vi "Demo Main.vi"() -> ()   [LabVIEW 2022 SP3]
uses:
  Logo.ctl
  C:/Users/Public/OneDrive/Desktop/PMT program/SampleCodeLabView/Kinesis_with_LabVIEW_Examples_LV12 - v3/Thorlabs.MotionControl.Controls.dll
  Kinesis_with_LabVIEW_Examples_LV12 - v3/Thorlabs.MotionControl.Controls.dll
  <vilib>/Utility/file.llb/Write Delimited Spreadsheet (string).vi
  <vilib>/Utility/file.llb/Write Delimited Spreadsheet (I64).vi
  <vilib>/Utility/file.llb/Write Delimited Spreadsheet (DBL).vi
  C:/Users/Public/OneDrive/Desktop/PMT program/SampleCodeLabView/Kinesis_with_LabVIEW_Examples_LV12 - v3/ThorLabs.MotionControl.KCube.DCServoCLI.dll
  Kinesis_with_LabVIEW_Examples_LV12 - v3/ThorLabs.MotionControl.KCube.DCServoCLI.dll
  <vilib>/Analysis/NI_AALBase.lvlib
panel:
  out "Polar Plot":picture
  in  "Wait to Start (ms)":i32
  in  "Laser Power (mW)":string="sample"
  in  "Sample Name":string="sample"
  in  "Save All Gate Data":bool
  out "ESD":i32=10000 caption="Steps\nAdded/Removed"
  in  "ES":i32 caption="Add /Remove \nSteps"
  out "Sweep Graph":u32[](graph)
  out "SM":i32 caption="Sweep\nMean"
  out "SN":i32 caption="Current Sweep Iteration"
  out "SND":i32 caption="Total No. of Sweeps"
  in  "Auto-Sweep":bool
  in  "P8":bool
  out "PC":i32 caption="Current \nPosition"
  out "WTD":i32=10000 caption="Wait Time (ms)\nRead Data"
  out "EPD":i32 caption="End Position\nRead Data"
  out "SPD":i32 caption="Start Position\nRead Data"
  out "SSD":i32 caption="Step Size\nRead Data"
  in  "SP":i32 caption="Start Position (degrees)\n Set Data"
  in  "WT":i32=10000 caption="Wait Time (ms)\n Set Data"
  in  "EP":i32 caption="End Position (degrees)\n Set Data"
  in  "P7":bool
  in  "SS":i32 caption="Step Size (degrees)\nSet Data"
  in  "Motor Controller\nSerialNumber":string="27261255"
  in  "KCubeDCServoControl":refnum<k24>(container)
  in  "Export":bool
  out "DB":u32[](array[numeric])
  out "OVL":bool caption="LED ON : Over Rang Data"
  out "OLD":i32
  out "GN":i32 caption="Gate Number"
  in  "Correction":bool=TRUE
  in  "Logo":T1
  out "Graph":u32[](graph)
  in  "Stop":bool
  in  "Start":bool
  in  "P6":bool
  out "RND":i32 caption="Read Number\nRead Data"
  in  "P5":bool
  in  "RN":i32=100 caption="Read Number\nSet Data"
  out "PowerD":i32 caption="Power\nRead Data"
  out "ITD":i32 caption="Internal Time\nRead Data"
  in  "P4":bool
  in  "P3":bool
  in  "IT":i32=100 caption="Internal Time\nSet Data"
  in  "P2":bool
  out "Handle Number":i32
  in  "P1":bool caption="Switch\nPower OFF/Power ON"
  in  "EXIT":bool
  # "pmt serial: 30430219"
  # "note: If you change angle between linear polarized light and half-wave plate by theta, the \npolarization after the wave plate is changed by twice theta. The code doesn't account for this.\nThis means we really need to go only to 180degrees, because at that point we have rotated the polarization by 360deg."
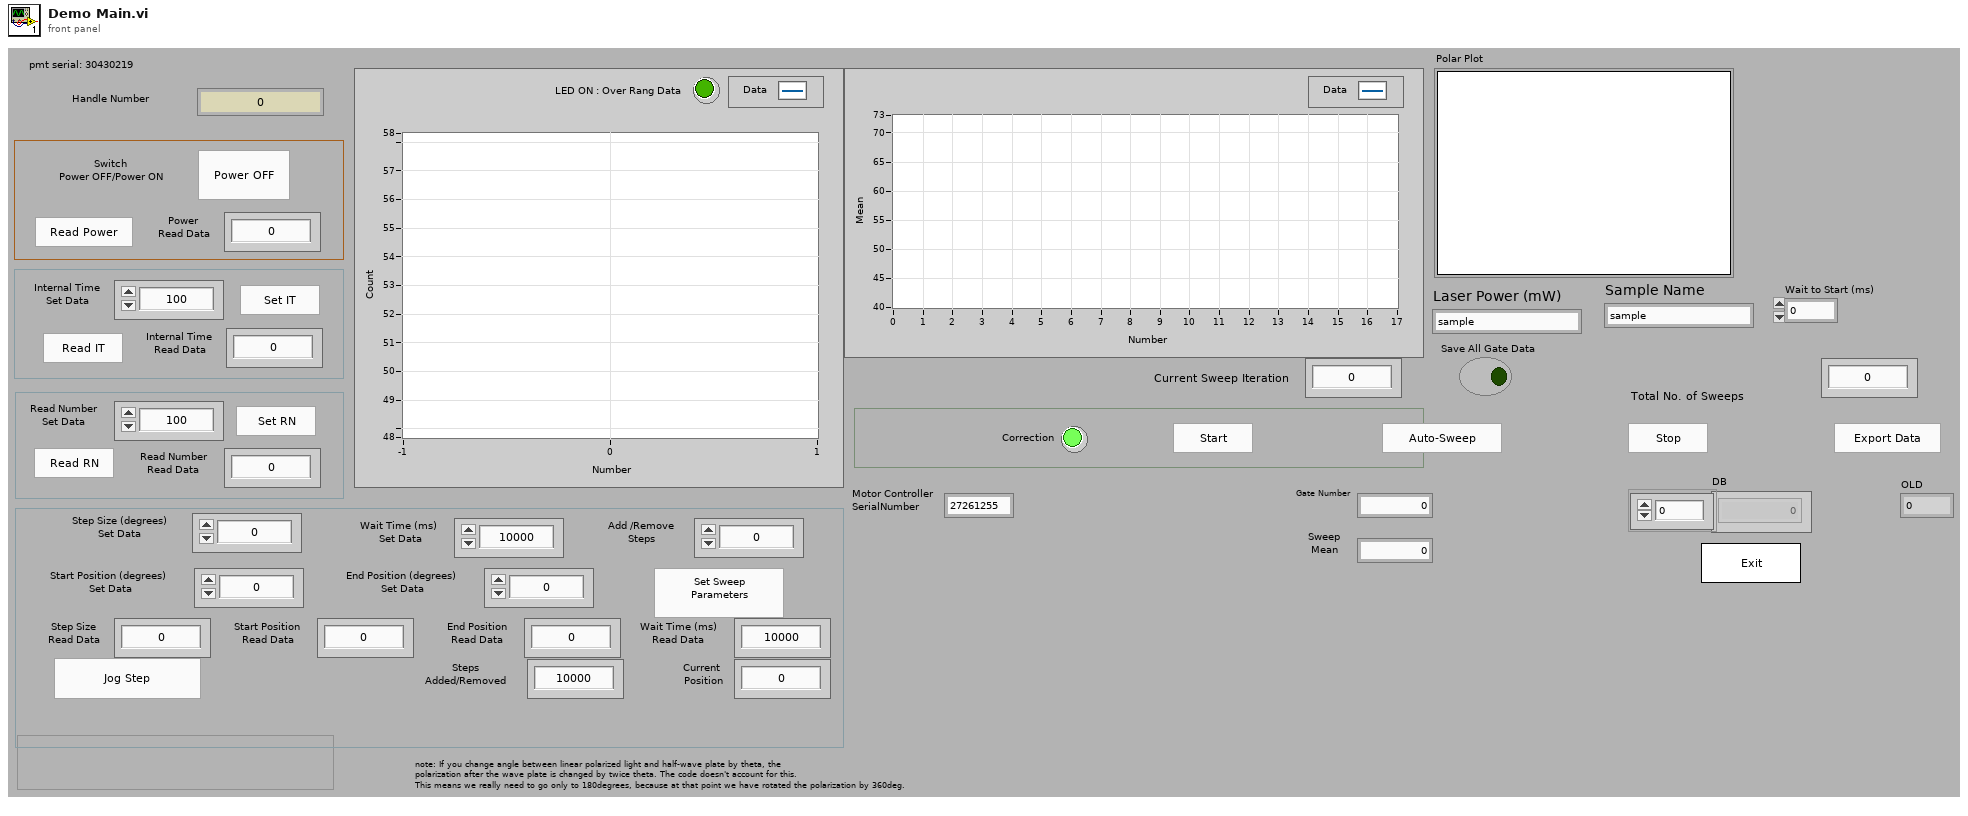
[diagram p1: front panel]
types:
  T1 = typedef "Logo.ctl" = bool
  T2 = enum8{"Enabled", "Disabled", "Disabled and Grayed Out"}
  T3 = typedef "LVBoundsTypeDef.ctl" = cluster{"Width":u32, "Height":u32}
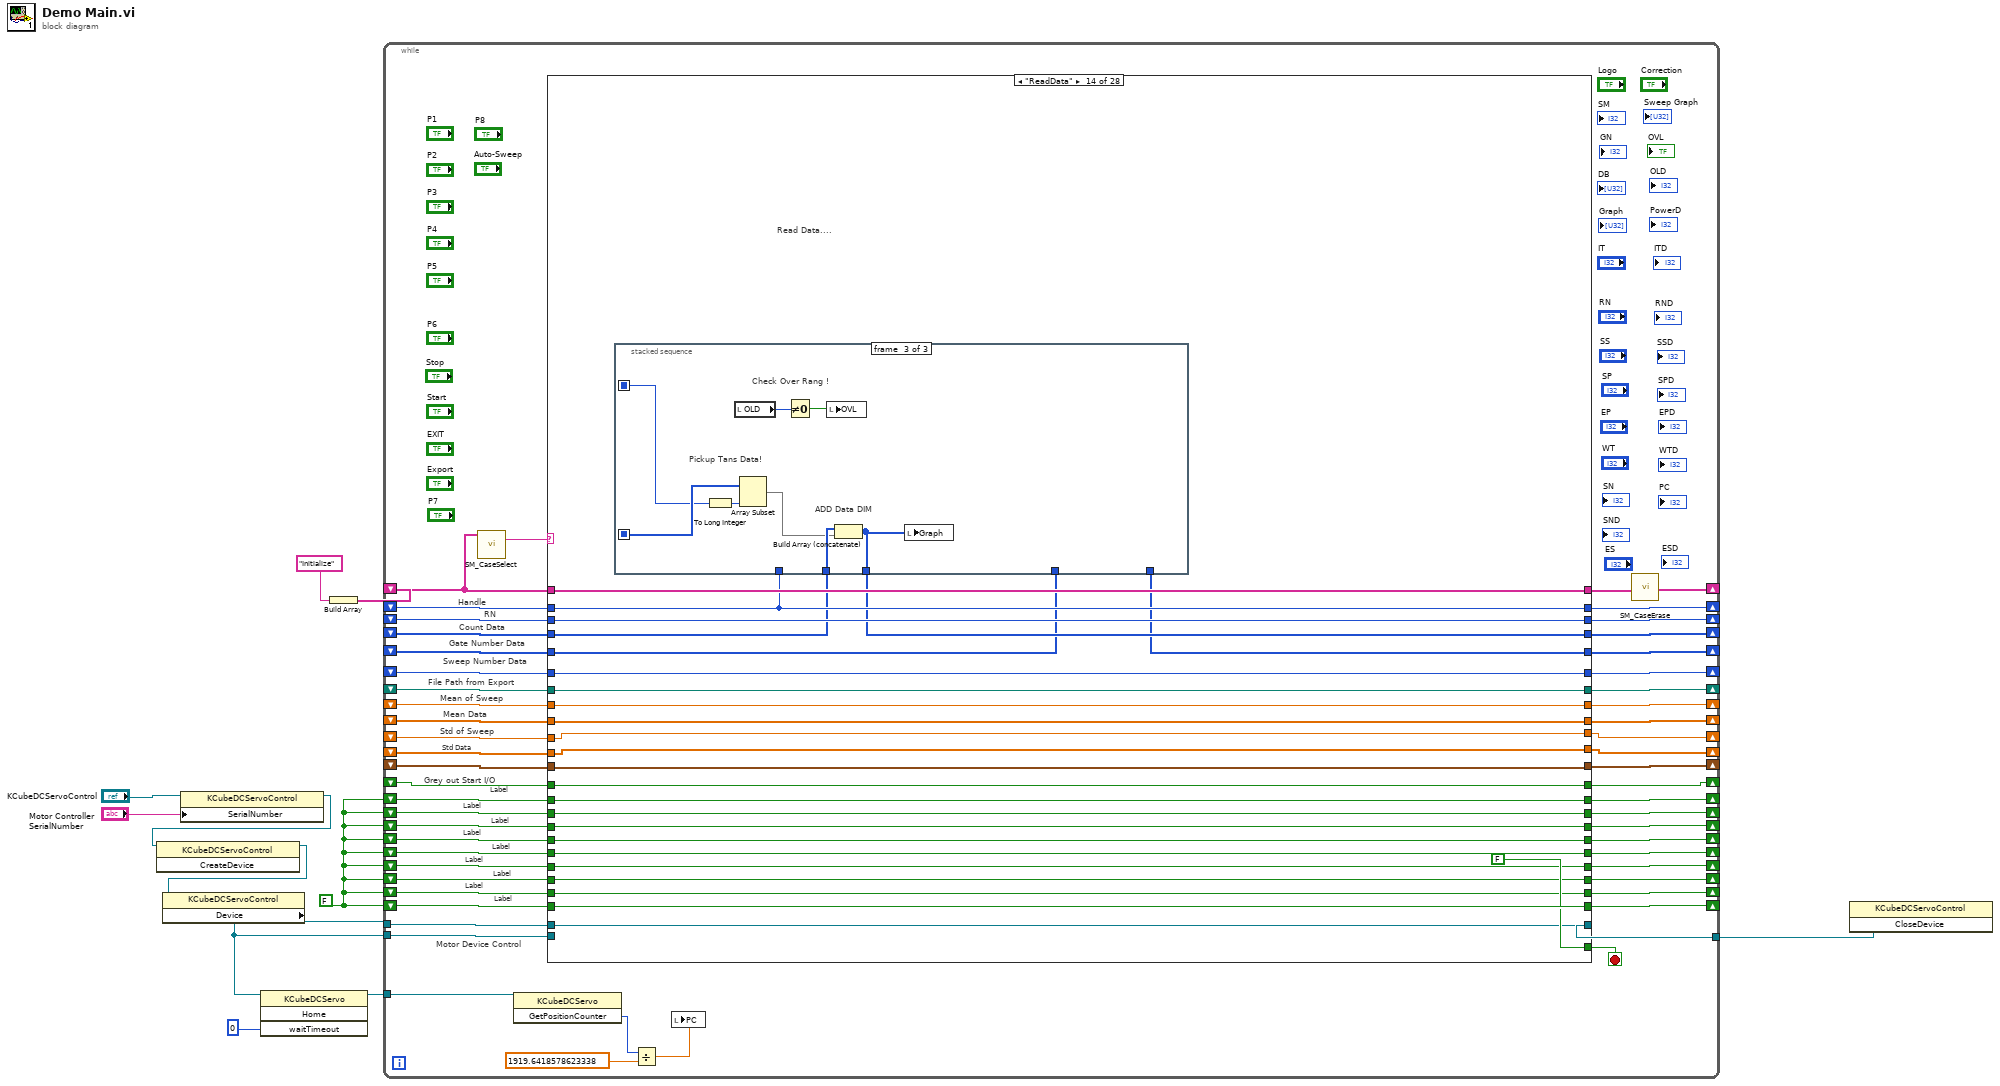
[diagram p0: block diagram]
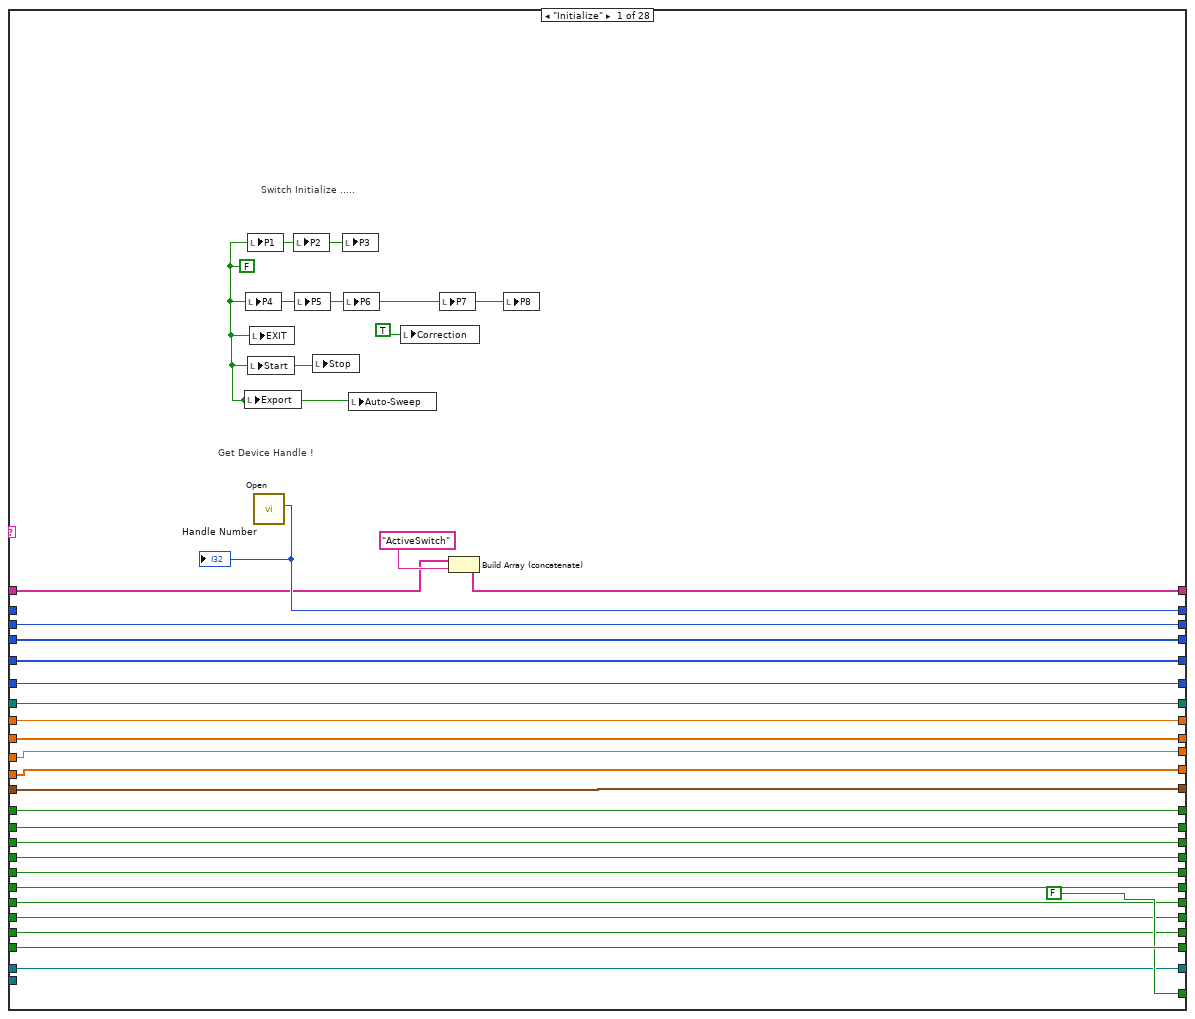
[diagram p2: hidden frame]
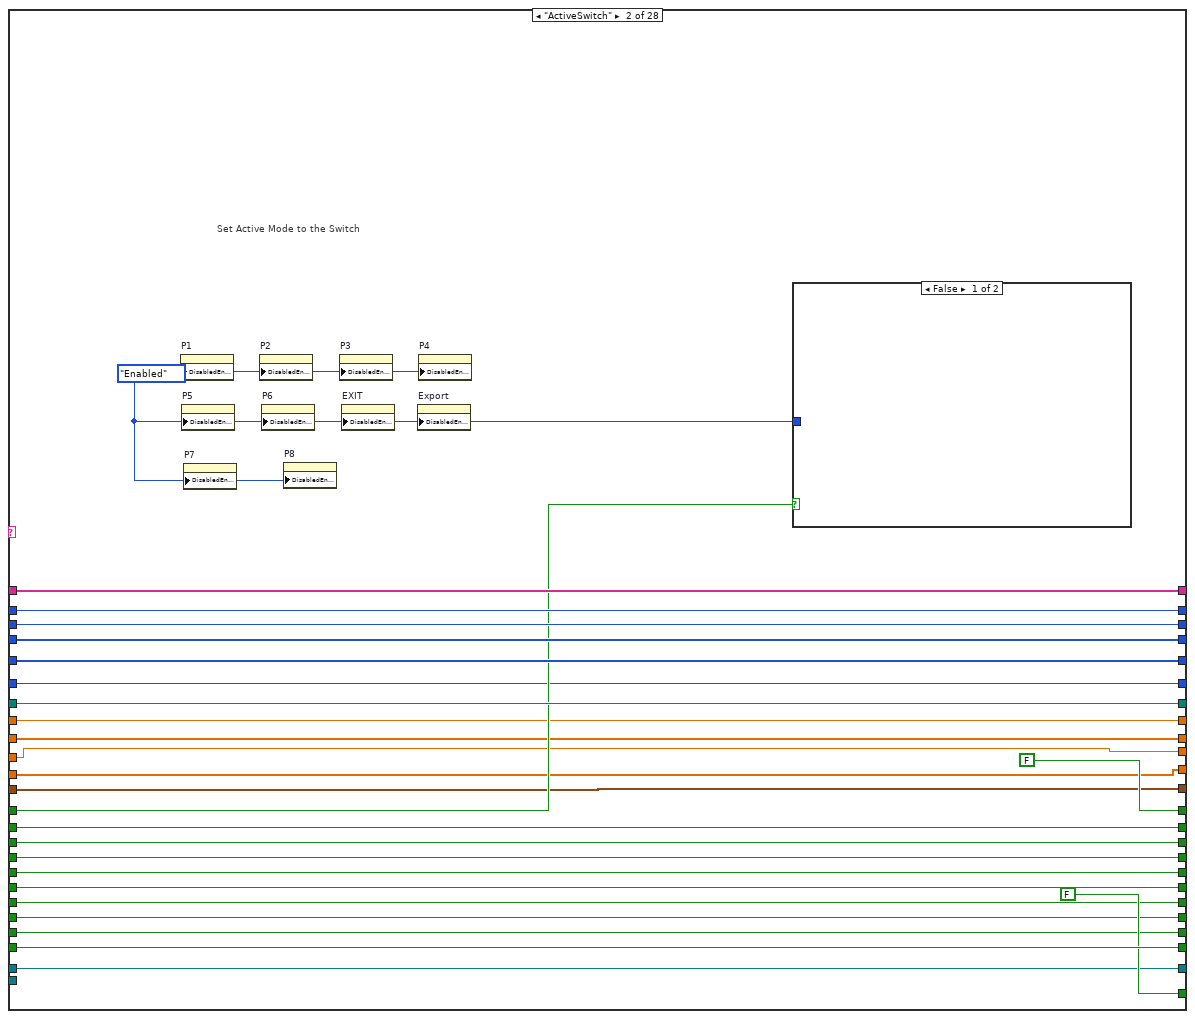
[diagram p3: hidden frame]
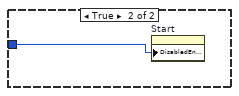
[diagram p4: hidden frame]
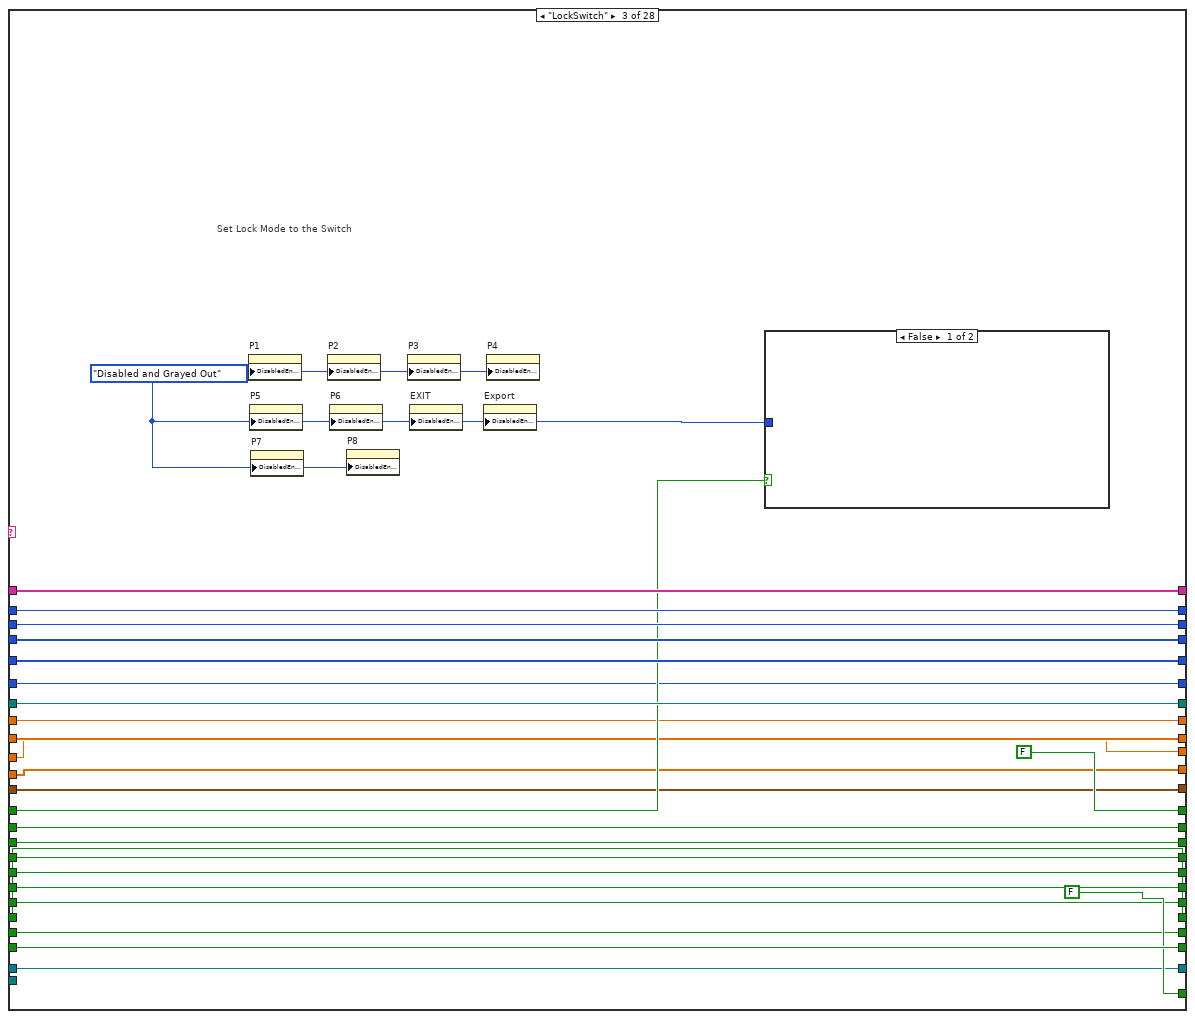
[diagram p5: hidden frame]
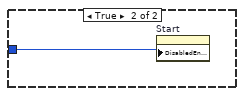
[diagram p6: hidden frame]
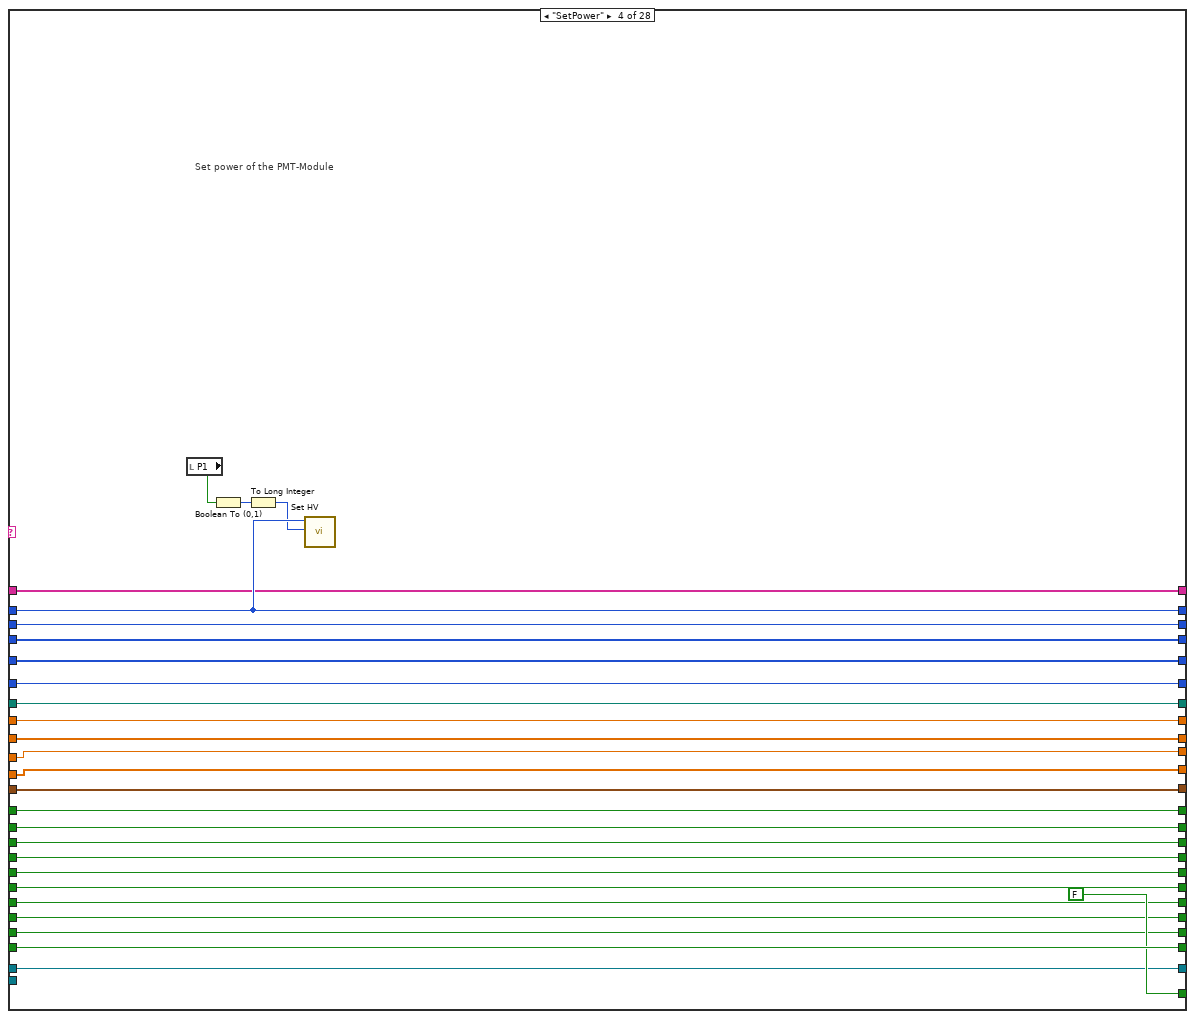
[diagram p7: hidden frame]
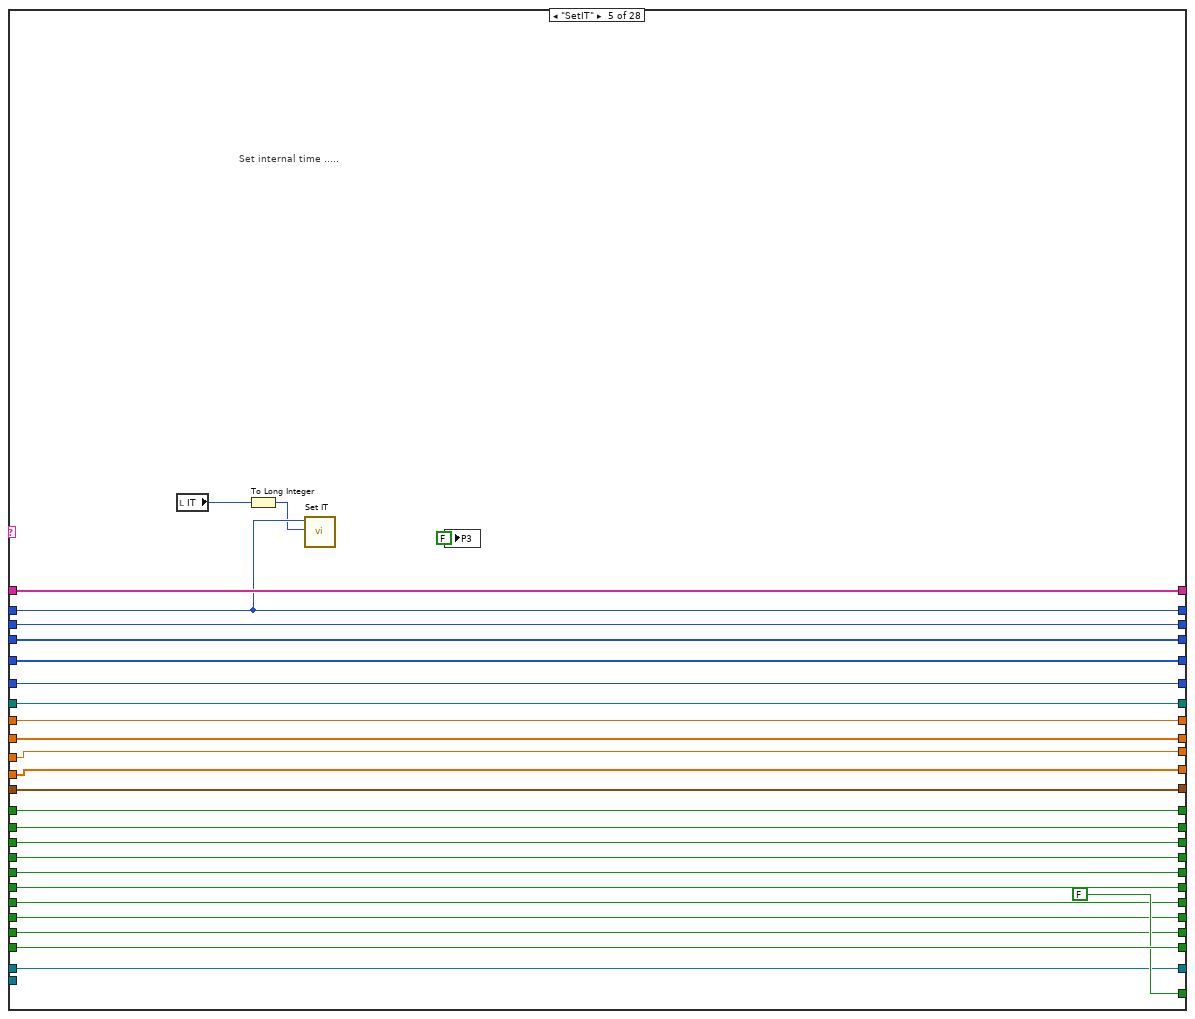
[diagram p8: hidden frame]
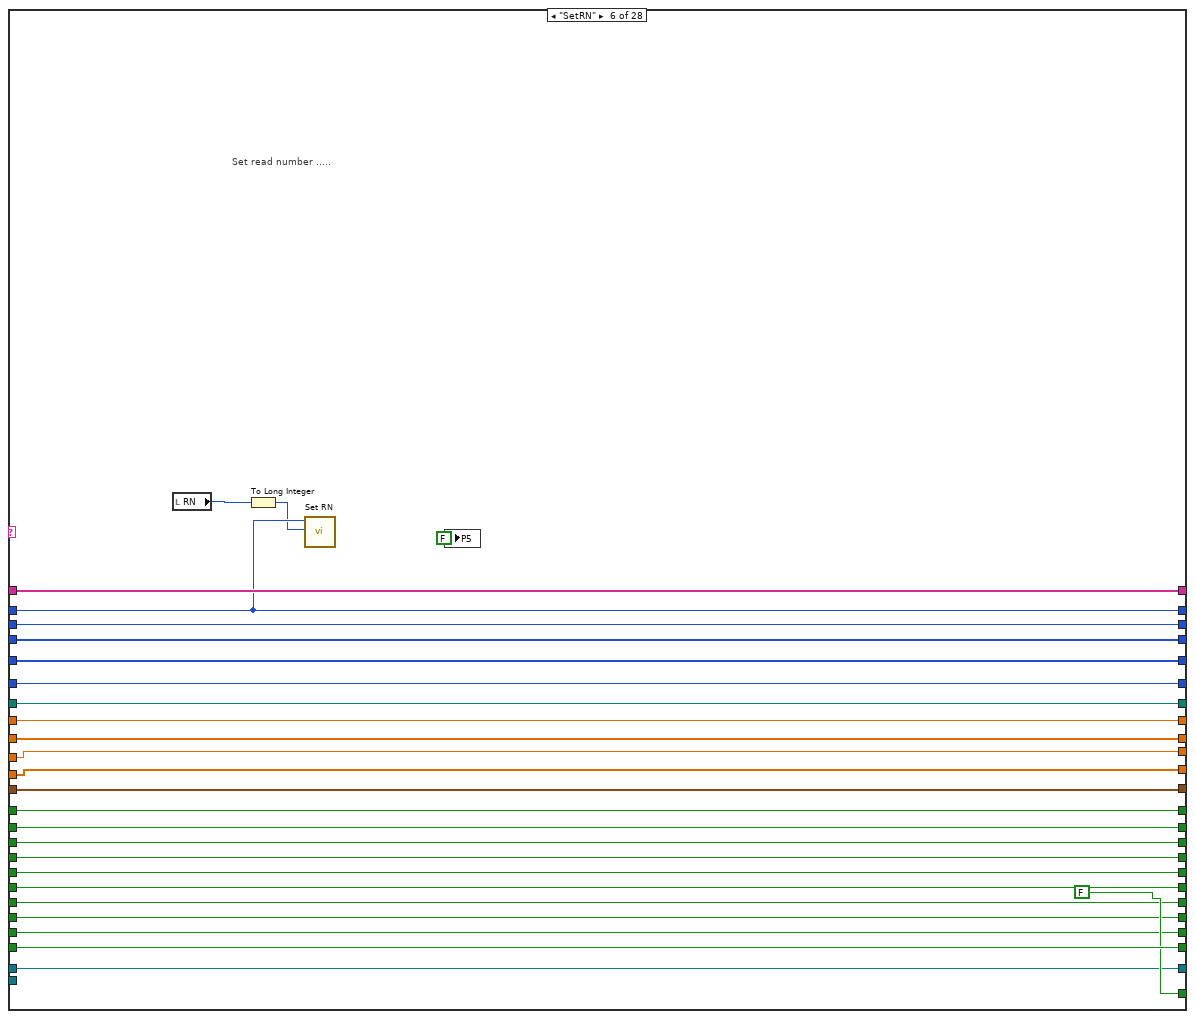
[diagram p9: hidden frame]
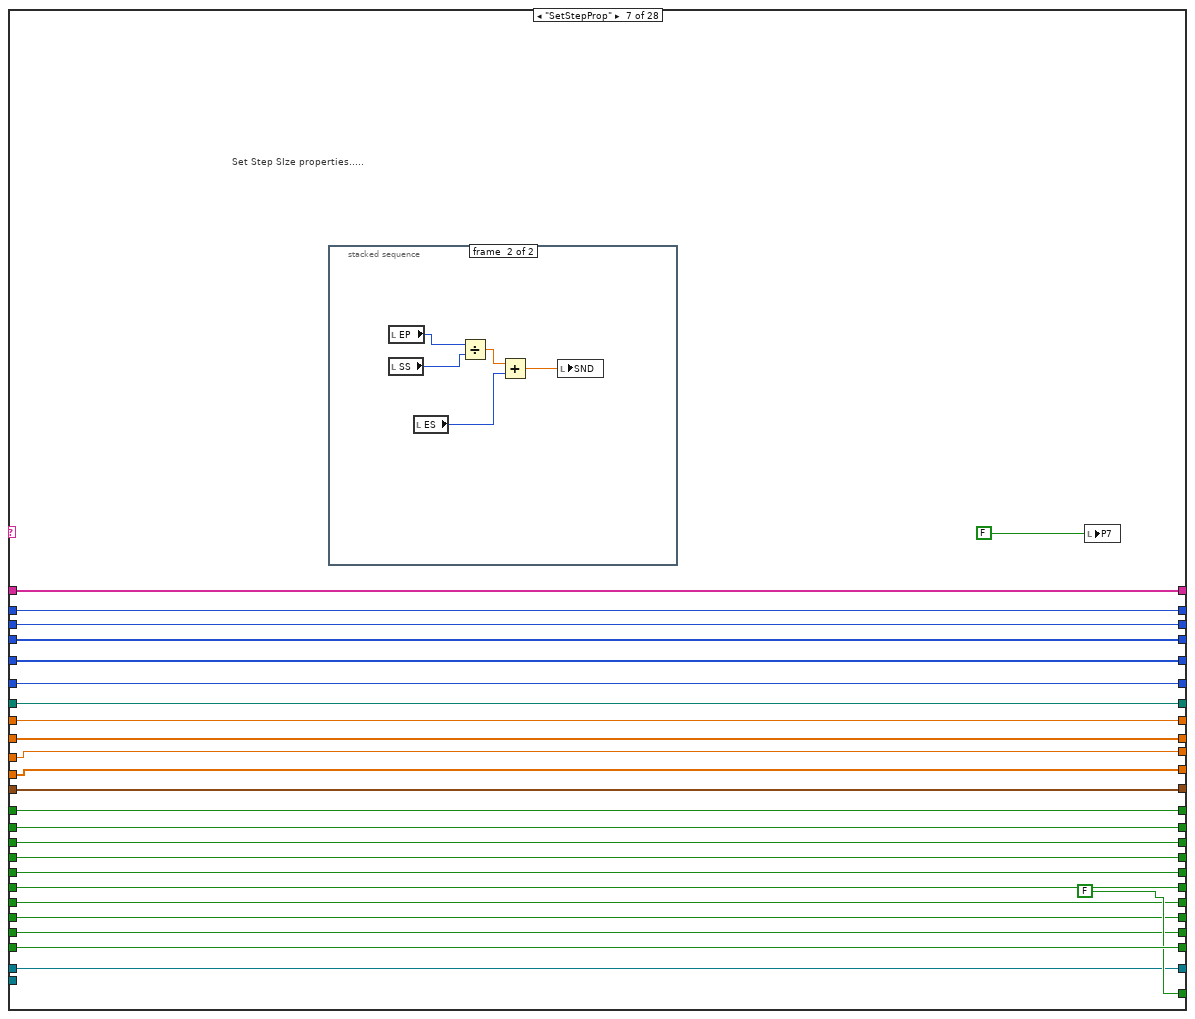
[diagram p10: hidden frame]
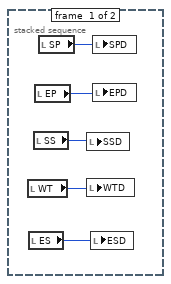
[diagram p11: hidden frame]
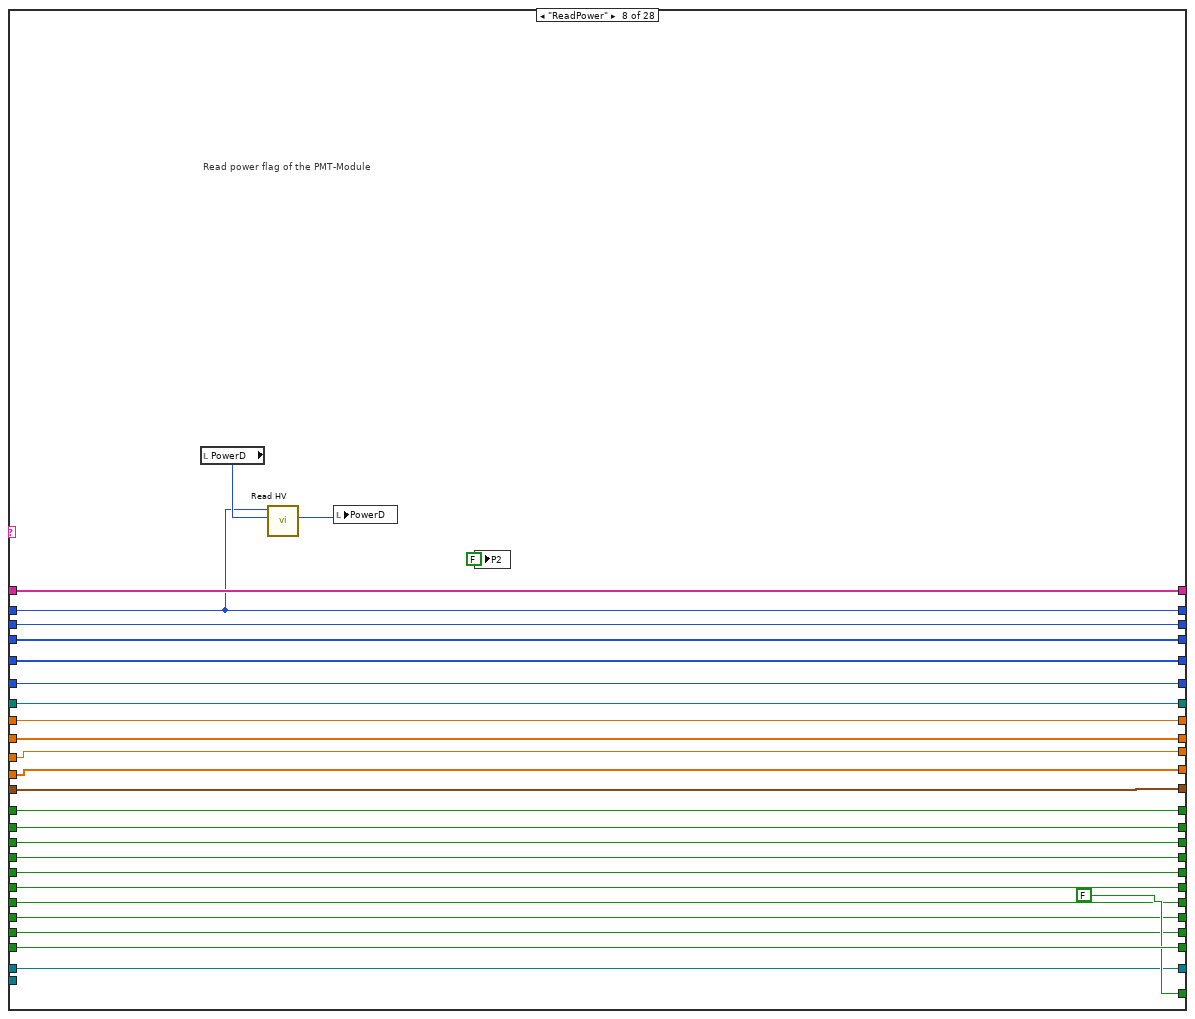
[diagram p12: hidden frame]
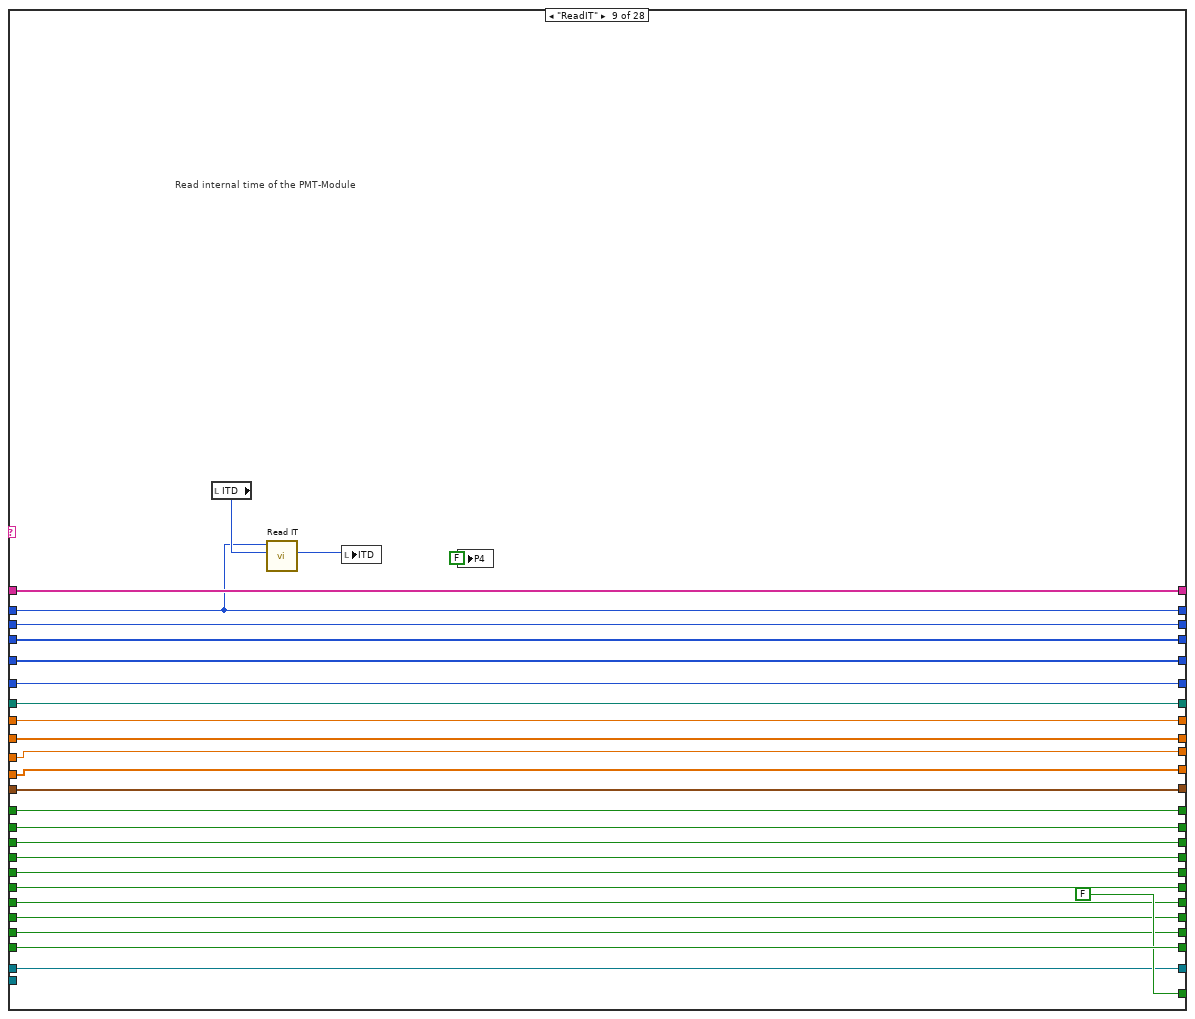
[diagram p13: hidden frame]
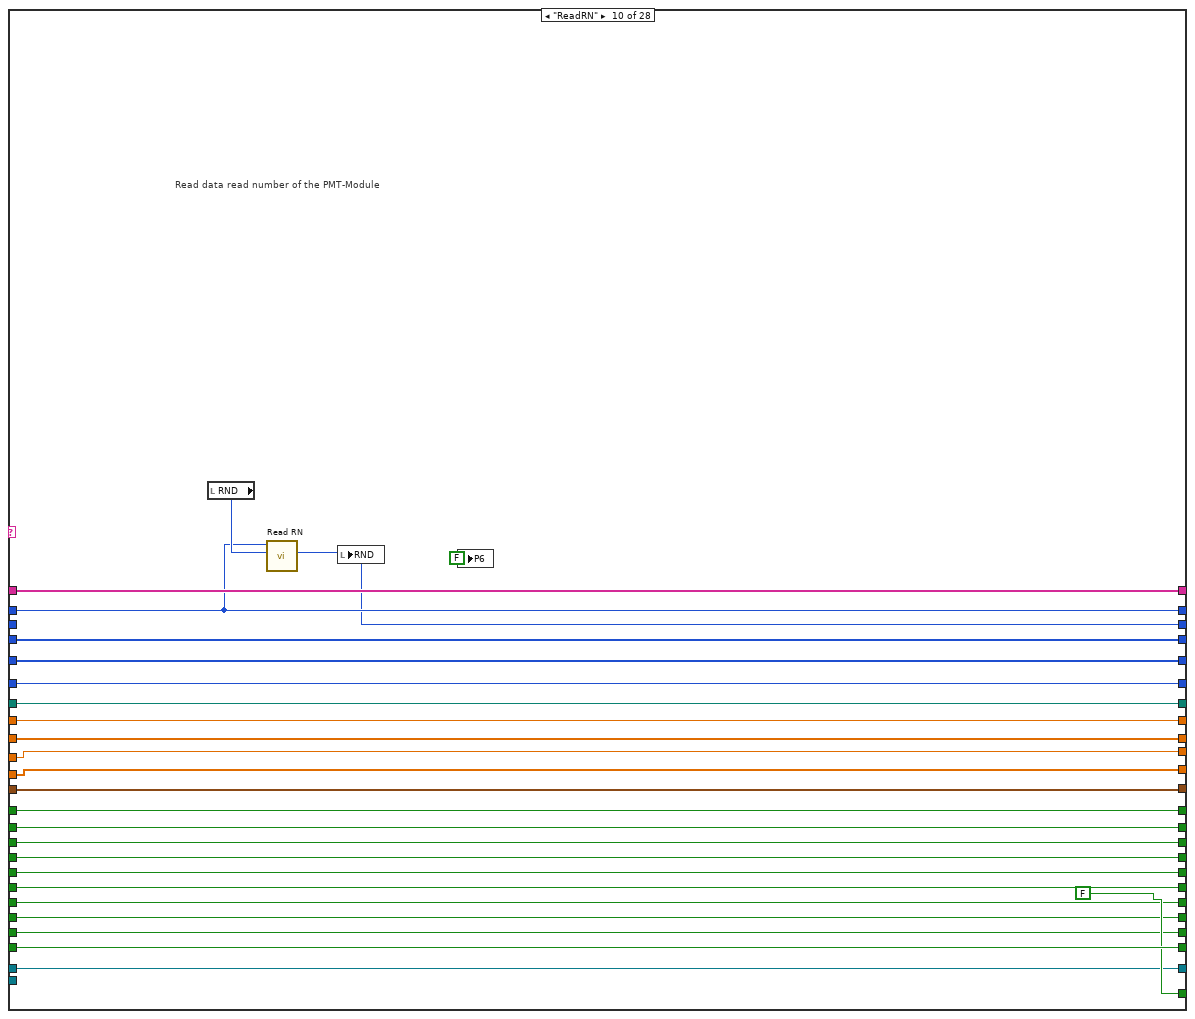
[diagram p14: hidden frame]
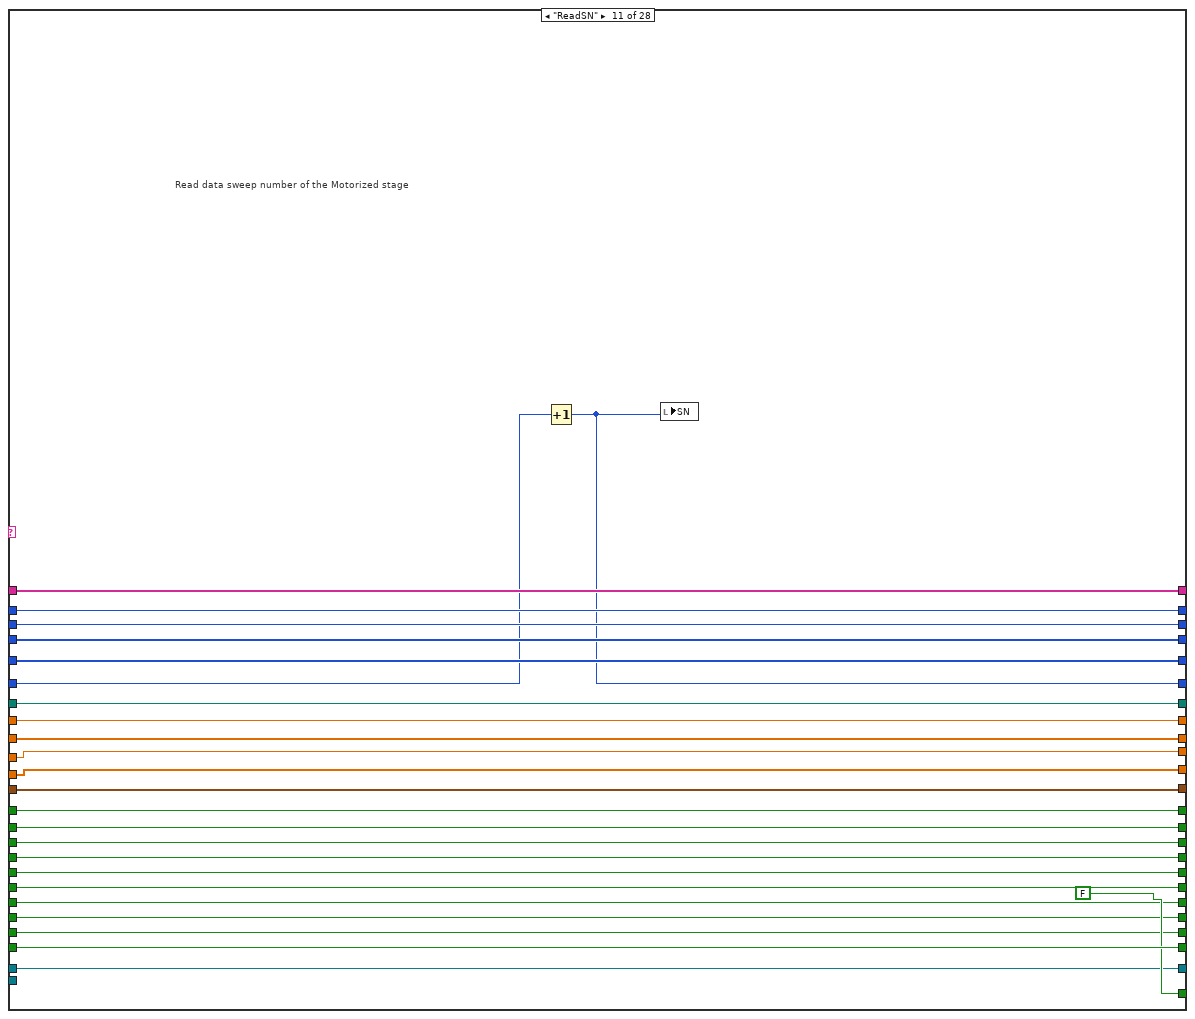
[diagram p15: hidden frame]
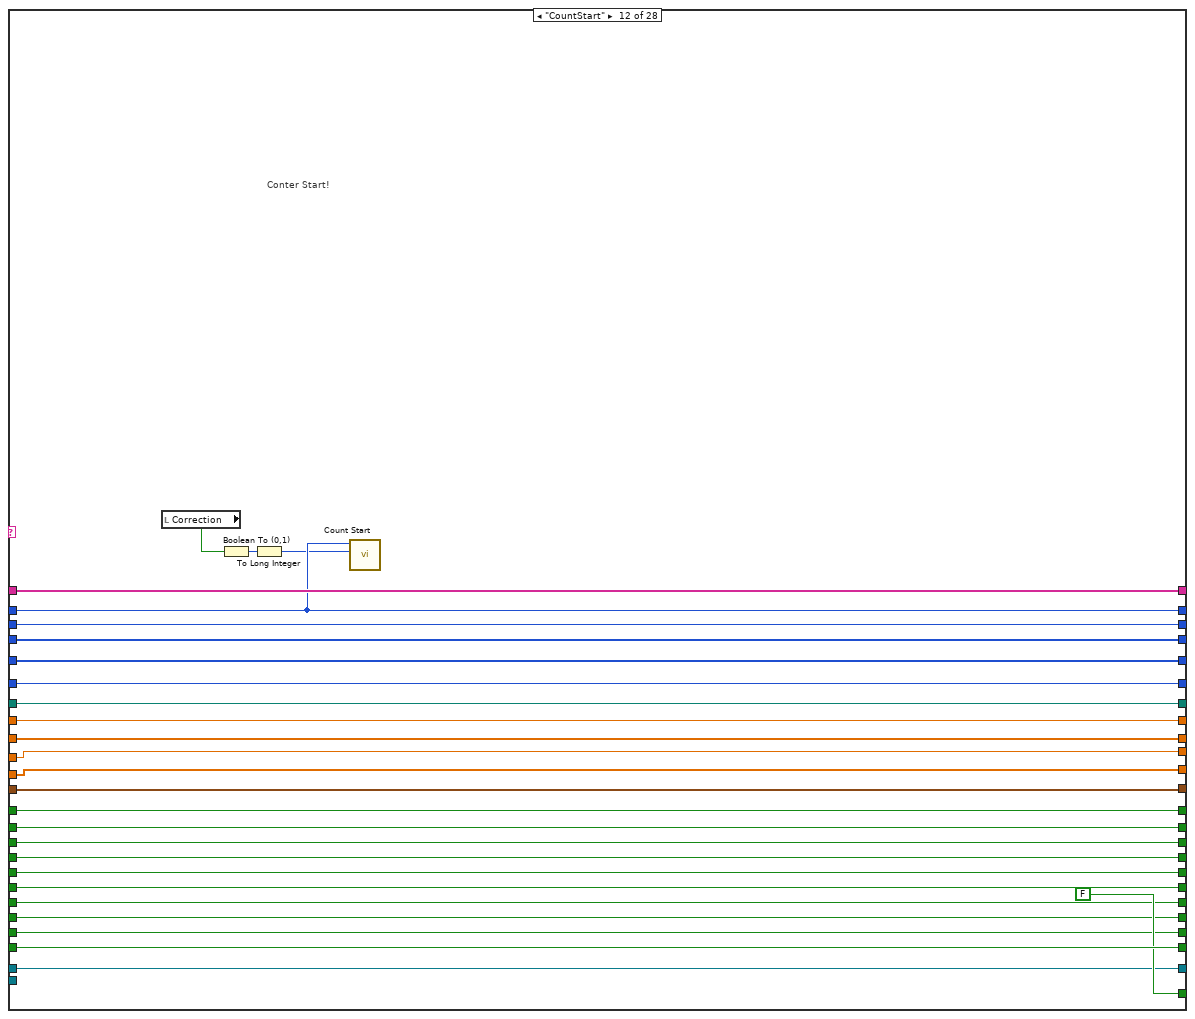
[diagram p16: hidden frame]
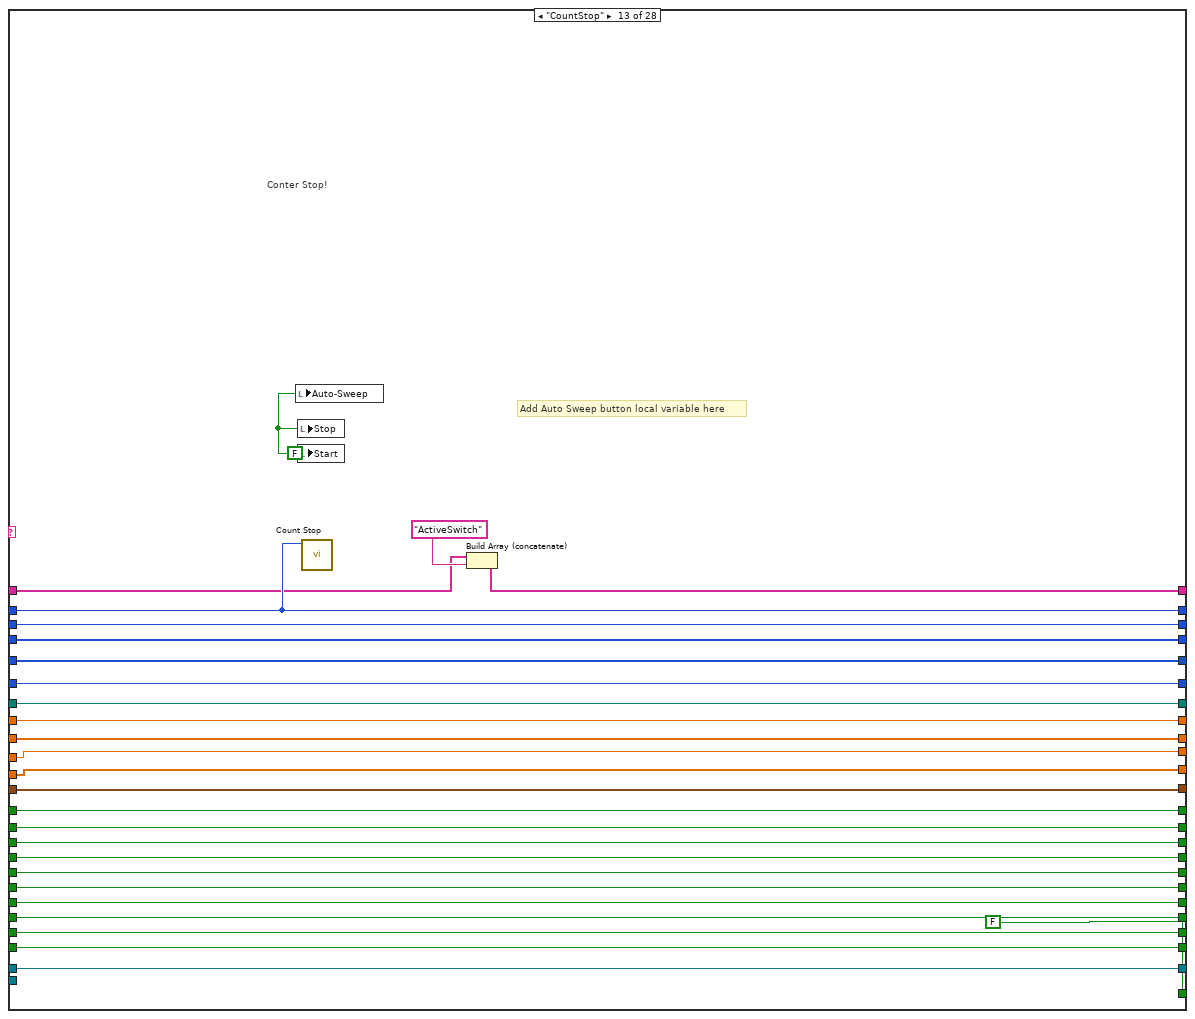
[diagram p17: hidden frame]
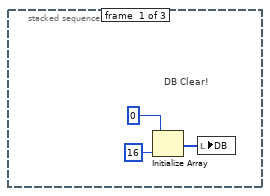
[diagram p18: hidden frame]
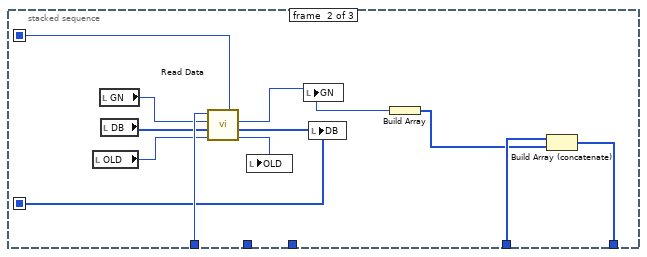
[diagram p19: hidden frame]
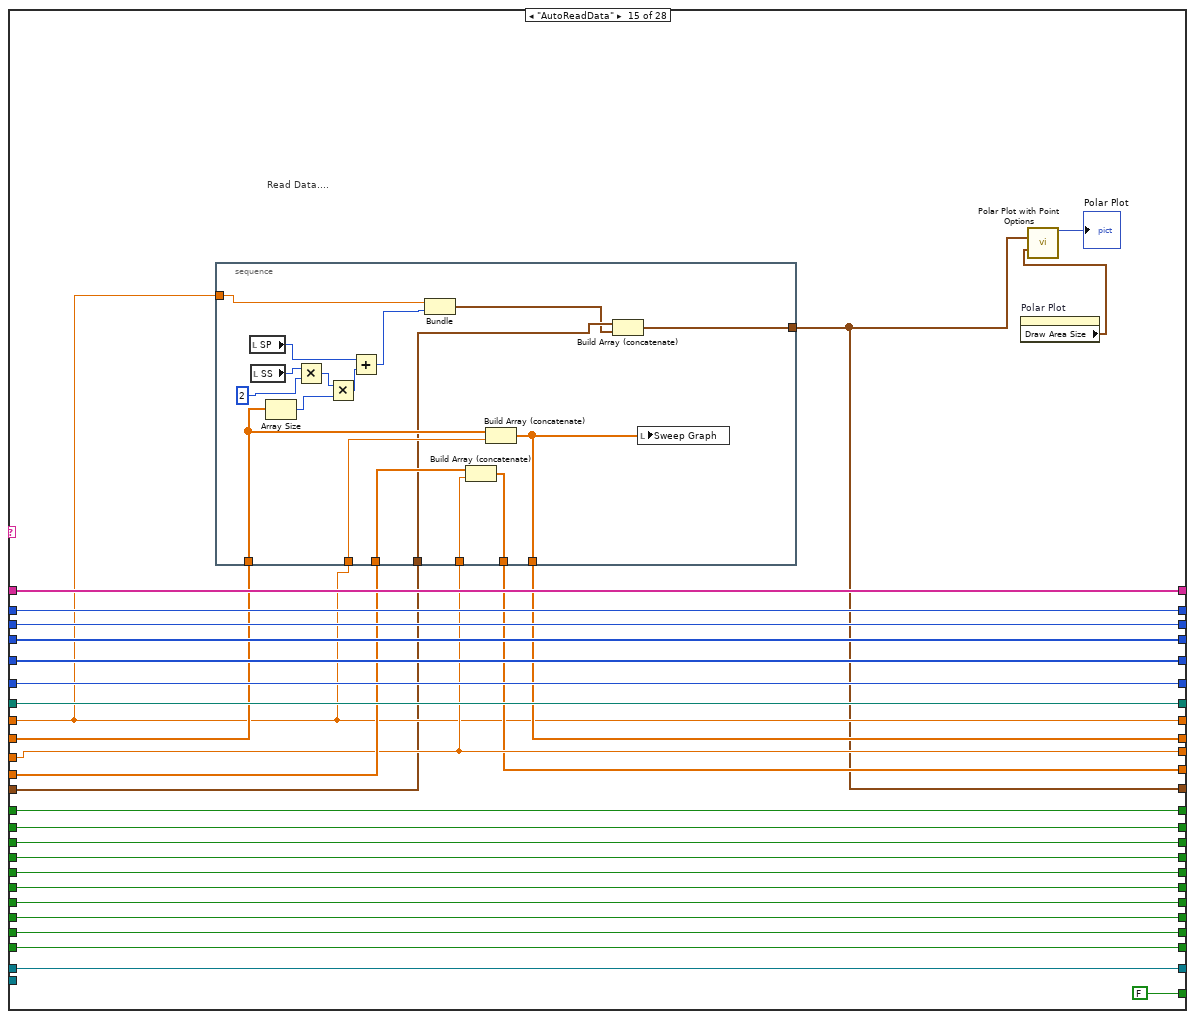
[diagram p20: hidden frame]
diagram:
  w10 = FALSE
  n1 = property class="KCubeDCServoControl"(reference="KCubeDCServoControl", "SerialNumber"="Motor Controller\nSerialNumber") -> (reference out=w9:refnum<k24>)  [unwired: 1 in, 1 out]
  n2 = invoke class="KCubeDCServoControl" method="CreateDevice"(reference=w9) -> (reference out=w2:refnum<k24>)  [unwired: 2 in, 2 out]
  n3 = property class="KCubeDCServoControl"(reference=w2) -> (reference out=w6:refnum<k24>, "Device"=w4:refnum<k24>)  [unwired: 1 in, 1 out]
  n4 = invoke class="KCubeDCServo" method="Home"(reference=w4, "waitTimeout"=0) -> (reference out=w3:refnum<k24>)  [unwired: 2 in, 3 out]
  n5 = Build Array("Initialize") -> (w11:string[])
  n6 = while {
    shift-right: [w49] -> _
    shift-left: w10 -> [w50]
    shift-right: [w51] -> _
    shift-left: w10 -> [w52]
    shift-right: [w53] -> _
    shift-left: w10 -> [w54]
    shift-right: [w55] -> _
    shift-left: w10 -> [w56]
    shift-right: [w57] -> _
    shift-left: _ -> [w58]
    shift-right: [w59] -> _
    shift-left: _ -> [w60]
    shift-right: [w61] -> _
    shift-left: _ -> [w62]
    shift-right: [w47] -> _
    shift-left: w10 -> [w48]
    shift-right: [w65] -> _
    shift-left: w10 -> [w66]
    shift-right: [w44] -> _
    shift-left: w11 -> [w63]
    shift-right: [w42] -> _
    shift-left: w10 -> [w43]
    shift-right: [w40] -> _
    shift-left: w10 -> [w41]
    shift-right: [w39] -> _
    shift-left: w10 -> [w38]
    tunnel: w6 -> [w35]
    tunnel: [w34] -> w7
    shift-right: [w37] -> _
    shift-left: _ -> [w36]
    tunnel: w4 -> [w33]
    shift-right: [w32] -> _
    shift-left: _ -> [w31]
    shift-right: [w30] -> _
    shift-left: _ -> [w29]
    tunnel: w3 -> [w28]
    shift-right: [w26] -> _
    shift-left: _ -> [w27]
    shift-right: [w25] -> _
    shift-left: _ -> [w24]
    shift-right: [w23] -> _
    shift-left: _ -> [w22]
    shift-right: [w18] -> _
    shift-left: _ -> [w19]
    shift-right: [w16] -> _
    shift-left: _ -> [w17]
    shift-right: [w14] -> _
    shift-left: _ -> [w13]
    stop <- w46 stop-if-true
    # "Std Data"
    # "Std of Sweep"
    # "Mean Data"
    # "Mean of Sweep"
    # "Sweep Number Data"
    # "Grey out Start I/O"
    # "Motor Device Control"
    # "File Path from Export"
    # "Gate Number Data"
    # "Label"
    # "Label"
    # "Label"
    # "Label"
    # "Label"
    # "Label"
    # "Label"
    # "Label"
    # "Label"
    # "Count Data"
    # "RN"
    # "Handle"
    n7 = call "SM_CaseSelect.vi"("Input"=w63) -> ("Case"=w64:string)  [unwired: 10 out]
    n8 = invoke class="KCubeDCServo" method="GetPositionCounter"(reference=w28) -> ("GetPositionCounter"=w20:i32)  [unwired: 2 in, 2 out]
    n9 = case shown="\"ReadData\"" w64 {
      selector: w64 -> [_ _ _ _ _ _ _ _ _ _ _ _ _ _ _ _ _ _ _ _ _ _ _ _ _ _ w1077 _]
      tunnel: w66 -> [w94 w120 w147 w175 w202 w229 w254 w291 w318 w344 w369 w396 w423 w449 w500 w548 w577 w620 w661 w733 w773 w860 w911 w936 w971 w1021 w1095 w1119]
      tunnel: [w94 w120 w147 w175 w202 w229 w254 w291 w318 w344 w369 w396 w423 w449 w500 w548 w577 w620 w661 w733 w773 w860 w911 w936 w971 w1021 w1095 w1119] -> w65
      tunnel: w63 -> [w80 w119 w146 w150 w201 w228 w253 w290 w317 w343 w368 w395 w409 w448 w499 w536 w555 w607 w649 w744 w784 w871 w903 w949 w984 w1009 w1094 w1118]
      tunnel: [w79 w119 w146 w150 w201 w228 w253 w290 w317 w343 w368 w395 w408 w448 w499 w535 w554 w608 w650 w744 w784 w871 w902 w949 w984 w1006 w1094 w1118] -> w45
      tunnel: w62 -> [_ w107 w134 w163 w189 w216 w241 w277 w304 w331 w357 w383 w411 w437 w488 w537 w566 w610 w651 w743 w783 w870 w923 w948 w983 w1020 w1093 w1106]
      tunnel: [w82 w107 w134 w163 w189 w216 w241 w277 w304 w331 w357 w383 w411 w437 w488 w537 w566 w610 w651 w743 w783 w870 w923 w948 w983 w1020 w1093 w1106] -> w61
      tunnel: w60 -> [w93 w118 w145 w174 w200 w227 w252 w289 w316 _ w350 w394 w422 w447 w498 w547 w576 w605 w647 w742 w782 w869 w922 w947 w982 w1019 w1092 w1117]
      tunnel: [w93 w118 w145 w174 w200 w227 w252 w289 w316 w329 w350 w394 w422 w447 w498 w547 w576 w605 w647 w742 w782 w869 w922 w947 w982 w1019 w1092 w1117] -> w59
      tunnel: w58 -> [w92 w117 w144 w173 w199 w226 w251 w288 w315 w342 w367 w393 w421 w436 w484 _ _ w601 w645 w718 w768 w850 w921 w946 w981 w1005 w1091 w1116]
      tunnel: [w92 w117 w144 w173 w199 w226 w251 w288 w315 w342 w367 w393 w421 w435 w484 w527 w564 w601 w645 w718 w768 w850 w921 w946 w981 w1005 w1091 w1116] -> w57
      tunnel: w56 -> [w91 w116 w143 w172 w198 w225 w250 w287 w314 w341 w366 w392 w420 w446 w497 w546 w575 w619 w660 w741 w781 w868 w919 w944 w979 w1018 w1090 w1115]
      tunnel: [w91 w116 w143 w172 w198 w225 w250 w287 w314 w341 w366 w392 w420 w446 w497 w546 w575 w619 w660 w741 w781 w868 w919 w944 w979 w1018 w1090 w1115] -> w55
      tunnel: w54 -> [w90 w115 w142 w171 w197 w224 w249 w286 w313 w340 w365 w391 w419 w445 w496 w545 w574 w618 w659 w740 w780 w867 w918 w943 w978 w1017 w1089 w1114]
      tunnel: [w90 w115 w142 w171 w197 w224 w249 w286 w313 w340 w365 w391 w419 w445 w496 w545 w574 w618 w659 w740 w780 w867 w918 w943 w978 w1017 w1089 w1114] -> w53
      tunnel: w52 -> [w89 w114 w141 w170 w196 w223 w248 w285 w312 w339 w364 w390 w418 w444 w495 w544 w573 w617 w658 w739 w779 w866 w917 w942 w977 w1016 w1088 w1113]
      tunnel: [w89 w114 w141 w170 w196 w223 w248 w285 w312 w339 w364 w390 w418 w444 w495 w544 w573 w617 w658 w739 w779 w866 w917 w942 w977 w1016 w1088 w1113] -> w51
      tunnel: w50 -> [w88 w113 w140 w169 w195 w222 w247 w284 w311 w338 w363 w389 w417 w443 w494 w543 w572 w616 w657 w738 w778 w865 w916 w941 w976 w1015 w1087 w1112]
      tunnel: [w88 w113 w140 w169 w195 w222 w247 w284 w311 w338 w363 w389 w417 w443 w494 w543 w572 w616 w657 w738 w778 w865 w916 w941 w976 w1015 w1087 w1112] -> w49
      tunnel: w48 -> [w87 w112 w139 w168 w194 w221 w246 w283 w310 w337 w362 w388 w416 w442 w493 w542 w571 w615 w656 w737 w777 w864 w915 w940 w975 w1014 w1086 w1111]
      tunnel: [w87 w112 w139 w168 w194 w221 w246 w283 w310 w337 w362 w388 w416 w442 w493 w542 w571 w615 w656 w737 w777 w864 w915 w940 w975 w1014 w1086 w1111] -> w47
      tunnel: [FALSE FALSE FALSE FALSE FALSE FALSE FALSE FALSE FALSE FALSE FALSE FALSE FALSE FALSE FALSE FALSE FALSE FALSE FALSE FALSE FALSE FALSE FALSE FALSE FALSE FALSE FALSE TRUE] -> w46
      tunnel: w43 -> [w83 w108 w135 w164 w190 w217 w242 w279 w306 w333 w358 w384 w412 w438 w489 w538 w567 w611 w652 w736 w776 w863 w914 w939 w974 w1010 w1082 w1107]
      tunnel: [w83 w108 w135 w164 w190 w217 w242 w279 w306 w333 w358 w384 w412 w438 w489 w538 w567 w611 w652 w736 w776 w863 w914 w939 w974 w1010 w1082 w1107] -> w42
      tunnel: w41 -> [w85 w110 w137 w166 w192 w219 w244 w281 w308 w335 w360 w386 w414 w440 w491 w540 w569 w613 w654 w735 w775 w862 w913 w938 w973 w1012 w1084 w1109]
      tunnel: [w85 w110 w137 w166 w192 w219 w244 w281 w308 w335 w360 w386 w414 w440 w491 w540 w569 w613 w654 w735 w775 w862 w913 w938 w973 w1012 w1084 w1109] -> w40
      tunnel: [w84 w109 w136 w165 w191 w218 w243 w280 w307 w334 w359 w385 w413 w439 w490 w539 w568 w612 w653 w734 w774 w861 w912 w937 w972 w1011 w1083 w1108] -> w39
      tunnel: w38 -> [w84 w109 w136 w165 w191 w218 w243 w280 w307 w334 w359 w385 w413 w439 w490 w539 w568 w612 w653 w734 w774 w861 w912 w937 w972 w1011 w1083 w1108]
      tunnel: [w78 w106 w133 w159 w185 w212 w240 w274 w301 w328 w356 w379 w407 w434 w483 w527 w564 w600 w644 w713 w754 w845 w920 w945 w980 w1004 w1076 w1105] -> w37
      tunnel: w36 -> [w78 w106 w133 w159 w185 w212 w240 w274 w301 w328 w356 w379 w407 w433 w483 _ _ w600 w644 w713 w754 w845 w920 w945 w980 w1004 w1076 w1105]
      tunnel: w35 -> [w77 w105 w132 w158 w184 w211 w239 w273 w300 w327 w355 w378 w406 w432 w487 w526 w563 w599 w643 w715 w766 w847 w910 w935 w970 w1003 w1075 w1104]
      tunnel: [w77 w105 w132 w158 w184 w211 w239 w273 w300 w327 w355 w378 w406 w432 w487 w526 w563 w599 w643 w715 w766 w847 w910 w935 w970 w1003 w1075 w1104] -> w34
      tunnel: w33 -> [_ _ _ _ _ _ _ _ _ _ _ _ _ _ _ _ _ _ _ _ _ _ _ w932 w967 _ _ _]
      tunnel: [w76 w104 w131 w157 w183 w210 w237 w272 w299 w326 w354 w377 w405 w431 w486 w525 w562 w598 w642 w706 w764 w832 w899 w933 w968 w1002 w1074 w1103] -> w32
      tunnel: w31 -> [w76 w104 w131 w157 w183 w210 w237 w272 w299 w326 w354 w377 w405 w431 w486 w525 w562 w598 w642 w706 w760 w831 _ w933 w968 w1002 w1074 w1103]
      tunnel: [w75 FALSE FALSE w156 w182 w209 w236 w271 w298 w325 w353 w376 w404 w430 w474 w524 TRUE w597 w641 w708 w763 w844 w908 w931 w966 w1001 w1073 w1102] -> w30
      tunnel: w29 -> [w75 w103 w130 w156 w182 w209 w236 w271 w298 w325 w353 w376 w404 w430 w474 w524 _ w597 _ w708 w763 w844 w908 w931 w966 w1001 w1073 w1102]
      tunnel: w27 -> [w73 w100 w127 w155 w181 w208 w235 w270 w297 w324 w348 w375 w403 w429 w485 w523 w560 w596 w640 w707 w759 w841 _ w927 w965 w1000 w1072 w1101]
      tunnel: [w73 w100 w127 w155 w181 w208 w235 w270 w297 w324 w349 w375 w403 w429 w485 w523 w560 w596 w640 w707 w759 w841 w900 w927 w965 w1000 w1072 w1101] -> w26
      tunnel: [w72 w99 w126 w154 w180 w207 w234 w269 w296 w323 w352 w374 w402 w428 w475 w522 w559 w595 w637 w705 w762 w836 w907 w929 w964 w999 w1071 w1100] -> w25
      tunnel: w24 -> [w72 w99 w126 w154 w180 w207 w234 w269 w296 w323 w352 w374 w402 w428 w475 w522 w559 w595 w637 w705 _ w836 w907 w929 w964 w999 w1071 w1100]
      tunnel: [w71 w98 w125 w153 w179 w206 w233 w268 w295 w322 w351 w373 w401 w427 w482 w521 w558 w594 w636 w704 w761 w840 w901 w928 w963 w998 w1070 w1099] -> w23
      tunnel: w22 -> [w71 w98 w125 w153 w179 w206 w233 w268 w295 w322 w351 w373 w401 w427 w481 w521 w558 w594 w636 w704 w761 w842 w901 w928 w963 w998 w1070 w1099]
      tunnel: w19 -> [w70 w97 w124 w152 w178 w205 w232 w267 w294 w321 w347 w372 w399 w426 w480 w520 w551 w593 w634 w703 w753 w838 w897 w926 w962 w997 w1069 w1098]
      tunnel: [w70 w97 w124 w152 w178 w205 w232 w267 w294 w321 w347 w372 w399 w426 w478 w520 w551 w593 w634 w703 w753 w839 w897 w926 w962 w997 w1069 w1098] -> w18
      tunnel: w17 -> [w69 w96 w123 w151 w177 w204 w231 w266 w293 w320 w346 w371 w398 w425 w479 w519 w550 w592 w633 w702 _ w835 w896 w925 w961 w996 w1068 w1097]
      tunnel: [w69 w96 w123 w151 w177 w204 w231 w266 w293 w320 w346 w371 w398 w425 w479 w519 w550 w592 w633 w702 w752 w835 w896 w925 w961 w996 w1068 w1097] -> w16
      tunnel: [w67 w95 w122 w149 w176 w203 w230 w265 w292 w319 w345 w370 w397 w424 w472 w518 w549 w591 w632 w701 w750 w818 w894 w924 w960 w995 w1067 w1096] -> w14
      tunnel: w13 -> [w67 w95 w122 w149 w176 w203 w230 w265 w292 w319 w345 w370 w397 w424 w473 w518 w549 w591 w632 w701 w750 _ w894 w924 w960 w995 w1067 w1096]
      frame "Initialize" {
        w74 = FALSE ("P1")
        # "Get Device Handle !"
        # "Switch Initialize ....."
        n10 = local write "Export"(w74) -> ()
        n11 = local write "P4"(w74) -> ()
        n12 = local write "P1"(w74) -> ()
        n13 = local write "Start"(w74) -> ()
        n14 = local write "EXIT"(w74) -> ()
        n15 = call "Open.vi"() -> ("Handle Number"=w82:i32)  [unwired: 10 in, 1 out]
        "Handle Number" <- w82
        n16 = local write "P2"(w74) -> ()
        n17 = local write "P5"(w74) -> ()
        n18 = local write "Stop"(w74) -> ()
        n19 = local write "P3"(w74) -> ()
        n20 = local write "P6"(w74) -> ()
        n21 = local write "Auto-Sweep"(w74) -> ()
        n22 = local write "Correction"(TRUE ("P1")) -> ()
        n23 = local write "P7"(w74) -> ()
        n24 = Build Array (concatenate)(w80, "ActiveSwitch") -> (w79:string[])
        n25 = local write "P8"(w74) -> ()
      }
      frame "ActiveSwitch" {
        w101 = T2."Enabled" ("無効")
        # "Set Active Mode to the Switch"
        n26 = property on="P1" class="Bool (strict)"("DisabledEnum"=w101) -> ()  [unwired: 2 in, 2 out]
        n27 = property on="P5" class="Bool (strict)"("DisabledEnum"=w101) -> ()  [unwired: 2 in, 2 out]
        n28 = property on="P7" class="Bool (strict)"("DisabledEnum"=w101) -> ()  [unwired: 2 in, 2 out]
        n29 = property on="P2" class="Bool (strict)"("DisabledEnum"=w101) -> ()  [unwired: 2 in, 2 out]
        n30 = property on="P6" class="Bool (strict)"("DisabledEnum"=w101) -> ()  [unwired: 2 in, 2 out]
        n31 = property on="P8" class="Bool (strict)"("DisabledEnum"=w101) -> ()  [unwired: 2 in, 2 out]
        n32 = property on="P3" class="Bool (strict)"("DisabledEnum"=w101) -> ()  [unwired: 2 in, 2 out]
        n33 = property on="EXIT" class="Bool (strict)"("DisabledEnum"=w101) -> ()  [unwired: 2 in, 2 out]
        n34 = property on="Export" class="Bool (strict)"("DisabledEnum"=w101) -> ()  [unwired: 2 in, 2 out]
        n35 = property on="P4" class="Bool (strict)"("DisabledEnum"=w101) -> ()  [unwired: 2 in, 2 out]
        n36 = case shown="False" w103 {
          tunnel: w101 -> [_ w121]
          frame False {
          }
          frame True {
            n37 = property on="Start" class="Bool (strict)"("DisabledEnum"=w121) -> ()  [unwired: 2 in, 2 out]
          }
        }
      }
      frame "LockSwitch" {
        w128 = T2."Disabled and Grayed Out" ("無効")
        # "Set Lock Mode to the Switch"
        n38 = property on="P1" class="Bool (strict)"("DisabledEnum"=w128) -> ()  [unwired: 2 in, 2 out]
        n39 = property on="P5" class="Bool (strict)"("DisabledEnum"=w128) -> ()  [unwired: 2 in, 2 out]
        n40 = property on="P7" class="Bool (strict)"("DisabledEnum"=w128) -> ()  [unwired: 2 in, 2 out]
        n41 = property on="P2" class="Bool (strict)"("DisabledEnum"=w128) -> ()  [unwired: 2 in, 2 out]
        n42 = property on="P6" class="Bool (strict)"("DisabledEnum"=w128) -> ()  [unwired: 2 in, 2 out]
        n43 = property on="P8" class="Bool (strict)"("DisabledEnum"=w128) -> ()  [unwired: 2 in, 2 out]
        n44 = property on="P3" class="Bool (strict)"("DisabledEnum"=w128) -> ()  [unwired: 2 in, 2 out]
        n45 = property on="EXIT" class="Bool (strict)"("DisabledEnum"=w128) -> ()  [unwired: 2 in, 2 out]
        n46 = property on="Export" class="Bool (strict)"("DisabledEnum"=w128) -> ()  [unwired: 2 in, 2 out]
        n47 = property on="P4" class="Bool (strict)"("DisabledEnum"=w128) -> ()  [unwired: 2 in, 2 out]
        n48 = case shown="False" w130 {
          tunnel: w128 -> [_ w148]
          frame False {
          }
          frame True {
            n49 = property on="Start" class="Bool (strict)"("DisabledEnum"=w148) -> ()  [unwired: 2 in, 2 out]
          }
        }
      }
      frame "SetPower" {
        # "Set power of the PMT-Module"
        n50 = local read "P1"() -> (w162:bool)
        n51 = Boolean To (0,1)(Boolean=w162) -> (0, 1=w161:i16)
        n52 = To Long Integer(number=w161) -> (32bit integer=w160:i32)
        n53 = call "Set HV.vi"("HV"=w160, "handle"=w163) -> ()  [unwired: 8 in, 2 out]
      }
      frame "SetIT" {
        # "Set internal time ....."
        n54 = local read "IT"() -> (w187:i32)
        n55 = To Long Integer(number=w187) -> (32bit integer=w188:i32)
        n56 = call "Set IT.vi"("IT"=w188, "handle"=w189) -> ()  [unwired: 8 in, 2 out]
        n57 = local write "P3"(FALSE ("P3")) -> ()
      }
      frame "SetRN" {
        # "Set read number ....."
        n58 = local read "RN"() -> (w214:i32)
        n59 = To Long Integer(number=w214) -> (32bit integer=w215:i32)
        n60 = call "Set RN.vi"("RN"=w215, "handle"=w216) -> ()  [unwired: 8 in, 2 out]
        n61 = local write "P5"(FALSE ("P3")) -> ()
      }
      frame "SetStepProp" {
        # "Set Step SIze properties....."
        n62 = stacked-sequence {
          frame #0 {
            n63 = local read "WT"() -> (w256:i32)
            n64 = local read "ES"() -> (w255:i32)
            n65 = local read "SS"() -> (w257:i32)
            n66 = local read "EP"() -> (w258:i32)
            n67 = local read "SP"() -> (w259:i32)
            n68 = local write "SSD"(w257) -> ()
            n69 = local write "WTD"(w256) -> ()
            n70 = local write "ESD"(w255) -> ()
            n71 = local write "SPD"(w259) -> ()
            n72 = local write "EPD"(w258) -> ()
          }
          frame #1 {
            n73 = local read "EP"() -> (w264:i32)
            n74 = local read "SS"() -> (w263:i32)
            n75 = local read "ES"() -> (w261:i32)
            n76 = Divide(x=w264, y=w263) -> (x/y=w262:dbl)
            n77 = Add(x=w262, y=w261) -> (x+y=w260:dbl)
            n78 = local write "SND"(w260) -> ()
          }
        }
        n79 = local write "P7"(FALSE) -> ()
      }
      frame "ReadPower" {
        # "Read power flag of the PMT-Module"
        n80 = local read "PowerD"() -> (w278:i32)
        n81 = call "Read HV.vi"("HV"=w278, "handle"=w277) -> ("HV out"=w276:i32)  [unwired: 7 in, 2 out]
        n82 = local write "PowerD"(w276) -> ()
        n83 = local write "P2"(FALSE ("P2")) -> ()
      }
      frame "ReadIT" {
        # "Read internal time of the PMT-Module"
        n84 = local read "ITD"() -> (w305:i32)
        n85 = call "Read IT.vi"("IT"=w305, "handle"=w304) -> ("IT out"=w303:i32)  [unwired: 7 in, 2 out]
        n86 = local write "ITD"(w303) -> ()
        n87 = local write "P4"(FALSE ("P4")) -> ()
      }
      frame "ReadRN" {
        # "Read data read number of the PMT-Module"
        n88 = local read "RND"() -> (w332:i32)
        n89 = call "Read RN.vi"("RN"=w332, "handle"=w331) -> ("RN out"=w329:i32)  [unwired: 7 in, 2 out]
        n90 = local write "RND"(w329) -> ()
        n91 = local write "P6"(FALSE ("P4")) -> ()
      }
      frame "ReadSN" {
        # "Read data sweep number of the Motorized stage"
        n92 = Increment(x=w348) -> (x+1=w349:i32)
        n93 = local write "SN"(w349) -> ()
      }
      frame "CountStart" {
        # "Conter Start!"
        n94 = local read "Correction"() -> (w380:bool)
        n95 = Boolean To (0,1)(Boolean=w380) -> (0, 1=w382:i16)
        n96 = To Long Integer(number=w382) -> (32bit integer=w381:i32)
        n97 = call "Count Start.vi"("Correction"=w381, "handle"=w383) -> ()  [unwired: 8 in, 2 out]
      }
      frame "CountStop" {
        w400 = FALSE ("Start")
        # "Add Auto Sweep button local variable here"
        # "Conter Stop!"
        n98 = local write "Auto-Sweep"(w400) -> ()
        n99 = local write "Stop"(w400) -> ()
        n100 = local write "Start"(w400) -> ()
        n101 = call "Count Stop.vi"("handle"=w411) -> ()  [unwired: 9 in, 2 out]
        n102 = Build Array (concatenate)(w409, "ActiveSwitch") -> (w408:string[])
      }
      frame "ReadData" {
        # "Read Data...."
        n103 = stacked-sequence {
          seq-local: [_ w458 _] -> [_ _ w468]
          seq-local: [_ w457 _] -> [_ _ w469]
          tunnel: w437 -> [_ w463 _]
          tunnel: w436 -> [_ _ w471]
          tunnel: [_ _ w470] -> w435
          tunnel: [_ w453 _] -> w434
          tunnel: w433 -> [_ w456 _]
          frame #0 {
            # "DB Clear!"
            n104 = Initialize Array(u32 0, 16 ("次元サイズ")) -> (w450:u32[])
            n105 = local write "DB"(w450) -> ()
          }
          frame #1 {
            n106 = local read "OLD"() -> (w460:i32)
            n107 = local read "GN"() -> (w462:i32)
            n108 = local read "DB"() -> (w461:u32[])
            n109 = call "Read Data.vi"("OLD"=w460, "DataBuf"=w461, "GateNum"=w462, "handle"=w463) -> ("OLD out"=w459:i32, "DataBuf out"=w457:u32[], "GateNum out"=w455:i32, "function return"=w458:u32)  [unwired: 3 in, 1 out]
            n110 = local write "OLD"(w459) -> ()
            n111 = local write "GN"(w455) -> ()
            n112 = local write "DB"(w457) -> ()
            n113 = Build Array(w455) -> (w454:i32[])
            n114 = Build Array (concatenate)(w456, w454) -> (w453:i32[])
          }
          frame #2 {
            # "Check Over Rang !"
            # "ADD Data DIM"
            # "Pickup Tans Data!"
            n115 = To Long Integer(number=w468) -> (32bit integer=w466:i32)
            n116 = local read "OLD"() -> (w465:i32)
            n117 = Array Subset(array=w469, length=w466) -> (w467:u32[])  [unwired: 1 in]
            n118 = Not Equal To 0?(x=w465) -> (x != 0?=w464:bool)
            n119 = local write "OVL"(w464) -> ()
            n120 = Build Array (concatenate)(w471, w467) -> (w470:u32[])
            n121 = local write "Graph"(w470) -> ()
          }
        }
      }
      frame "AutoReadData" {
        # "Read Data...."
        n122 = stacked-sequence {
          tunnel: w475 -> [w517]
          tunnel: [w516] -> w482
          tunnel: w481 -> [w511]
          tunnel: w480 -> [w515]
          tunnel: w479 -> [w514]
          tunnel: [w513] -> w478
          tunnel: w475 -> [w512]
          tunnel: w473 -> [w506]
          tunnel: [w504] -> w472
          frame #0 {
            n123 = local read "SP"() -> (w508:i32)
            n124 = local read "SS"() -> (w503:i32)
            n125 = Array Size(array=w511) -> (size(s)=w510:i32)
            n126 = Multiply(x=w503, y=2) -> (x*y=w502:i32)
            n127 = Multiply(x=w502, y=w510) -> (x*y=w509:i32)
            n128 = Add(x=w508, y=w509) -> (x+y=w507:i32)
            n129 = Bundle("mean"=w512, w507) -> (w505:cluster{"mean":dbl, i32})  [unwired: 1 in]
            n130 = Build Array (concatenate)(w515, w514) -> (w513:dbl[])
            n131 = Build Array (concatenate)(w511, w517) -> (w516:dbl[])
            n132 = Build Array (concatenate)(w506, w505) -> (w504:cluster{"mean":dbl, i32}[])
            n133 = local write "Sweep Graph"(w516) -> ()
          }
        }
        n134 = property on="Polar Plot" class="Pict"() -> ("Draw Area Size"=w477:T3)  [unwired: 2 in, 2 out]
        n135 = call <vilib>:"Polar Plot with Point Options.vi"("data array [mag, phase (deg)]"=w472, "dimensions (w,h)"=w477) -> ("new picture"=→"Polar Plot":picture)  [unwired: 13 in]
      }
      frame "CountInit" {
        w529 = 0
        # "Auto"
        # "Clear Data DIM !"
        n136 = Initialize Array(w529, w529) -> (w527:i32[])
        n137 = Build Array("LockSwitch", "ReadRN", "CountStart", "ReadData", "CheckNumber") -> (w530:string[])
        n138 = Build Array (concatenate)(w536, w530) -> (w535:string[])
      }
      frame "AutoCount|nit!" {
        w565 = 0
        # "Clear Data DIM !"
        n139 = local read "SND"() -> (w552:i32)
        n140 = local read "SN"() -> (w557:i32)
        n141 = Increment(x=w552) -> (x+1=w553:i32)
        n142 = Initialize Array(w565, w565) -> (w564:i32[])
        n143 = Less?(x=w557, y=w553) -> (x < y?=w556:bool)
        n144 = case shown="True" w556 {
          tunnel: w555 -> [w581 w584]
          tunnel: [w579 w583] -> w554
          frame False {
            n145 = Build Array("AutoReadData", "AutoCheckNumber") -> (w580:string[])
            n146 = Build Array (concatenate)(w581, w580) -> (w579:string[])
          }
          frame True {
            n147 = Build Array("LockSwitch", "ReadRN", "CountStart", "ReadData", "AutoCheckNumber") -> (w590:string[])
            n148 = Build Array (concatenate)(w584, w590) -> (w583:string[])
          }
        }
      }
      frame "CheckNumber" {
        # "Add append"
        # "Add Case Strucutre outside\nsimilar to GN,"
        # "Check RN and Data lenbgth,Stop Switch ......"
        n149 = local read "Stop"() -> (w602:bool)
        n150 = local read "GN"() -> (w603:i32)
        n151 = Decrement(x=w605) -> (x-1=w604:i32)
        n152 = Less?(x=w603, y=w604) -> (x < y?=w609:bool)
        n153 = case shown="True" w609 {
          tunnel: [w624 w626] -> w606
          tunnel: w602 -> [_ w625]
          frame False {
            # "\"MotorJog\"; here"
            # "Move \"Active Swith\" to False Condition of Position Number"
            # "Add \"AutoExport Run\" here"
            n154 = local write "Start"(FALSE ("Start")) -> ()
            n155 = Build Array("CountStop", "ActiveSwitch") -> (w624:string[])
          }
          frame True {
            n156 = case shown="True" w625 {
              tunnel: [w628 w630] -> w626
              frame False {
                n157 = Build Array("ReadData", "CheckNumber") -> (w628:string[])
              }
              frame True {
                n158 = Build Array("CountStop") -> (w630:string[])
              }
            }
          }
        }
        n159 = Build Array (concatenate)(w607, w606) -> (w608:string[])
      }
      frame "AutoCheckNumber" {
        # "Add append"
        # "Add Case Strucutre outside\nsimilar to GN,"
        # "Check RN and Data lenbgth,Stop Switch ......"
        n160 = local read "Stop"() -> (w646:bool)
        n161 = local read "SND"() -> (w635:i32)
        n162 = local read "SN"() -> (w639:i32)
        n163 = Less?(x=w639, y=w635) -> (x < y?=w638:bool)
        n164 = case shown="False" w638 {
          tunnel: [w663 w673] -> w648
          tunnel: w647 -> [_ w672]
          tunnel: w646 -> [_ w669]
          tunnel: [TRUE w668] -> w641
          frame False {
            w667 = FALSE ("Start")
            n165 = local write "Auto-Sweep"(w667) -> ()
            n166 = local write "Start"(w667) -> ()
            n167 = Build Array("CountStop", "AutoExportSweep", "ActiveSwitch") -> (w663:string[])
          }
          frame True {
            n168 = local read "GN"() -> (w670:i32)
            n169 = Decrement(x=w672) -> (x-1=w671:i32)
            n170 = Less?(x=w670, y=w671) -> (x < y?=w674:bool)
            n171 = case shown="False" w674 {
              tunnel: [w676 w692] -> w673
              tunnel: w669 -> [w677 w691]
              tunnel: [w675 w690] -> w668
              frame False {
                # "\"MotorJog\"; here"
                # "Move \"Active Swith\" to False Condition of Position Number"
                # "Add \"AutoExport Run\" here"
                n172 = case shown="False" w677 {
                  tunnel: [w683 w688] -> w676
                  tunnel: [FALSE TRUE] -> w675
                  frame False {
                    n173 = Build Array("CountStop", "AutoExportRun", "AutoReadData", "ReadSN", "MotorJog", "AutoCount|nit!") -> (w683:string[])
                  }
                  frame True {
                    n174 = local write "Auto-Sweep"(TRUE) -> ()
                    n175 = Build Array("CountStop") -> (w688:string[])
                  }
                }
              }
              frame True {
                n176 = case shown="False" w691 {
                  tunnel: [w695 w699] -> w692
                  tunnel: [FALSE TRUE] -> w690
                  frame False {
                    n177 = Build Array("ReadData", "AutoCheckNumber") -> (w695:string[])
                  }
                  frame True {
                    n178 = Build Array("CountStop") -> (w699:string[])
                    n179 = local write "Auto-Sweep"(TRUE) -> ()
                  }
                }
              }
            }
          }
        }
        n180 = Build Array (concatenate)(w649, w648) -> (w650:string[])
      }
      frame "Export" {
        # "For Auto Export also add mean waveform"
        # "Get mean Data into 1D array Shift register for waveform"
        # "Gate Number is just number of count measurements"
        # "time...using array size"
        # "time...using array size"
        n181 = Array Size(array=w718) -> (size(s)=w730:i32)
        n182 = for {
          N: w730 -> [_]
          tunnel: [w745] -> w717 mode=indexing
          i -> [w747]
          n183 = local read "ITD"() -> (w749:i32)
          n184 = Add(x=1, y=w747) -> (x+y=w748:i32)
          n185 = Multiply(x=w749, y=w748) -> (x*y=w745:i32)
        }
        n186 = call <vilib>:"Std Deviation and Variance.vi"("X"=w718) -> ("mean"=w711:dbl, "standard deviation"=w710:dbl)  [unwired: 1 in, 1 out]
        n187 = Build Array(w711, w710) -> (w709:dbl[])
        n188 = Build Array(w713, w717, w718) -> (w728:u32[][])
        n189 = call-poly <vilib>:"Write Delimited Spreadsheet.vi"("1D data"=string[] ["Gate  No.", "Time [ms]", "Counts"], "append to file? (new file:F)"=FALSE, "transpose? (no:F)"=FALSE) -> ("new file path (Not A Path if cancelled)"=w727:path)  [unwired: 11 in, 1 out]
        n190 = call-poly <vilib>:"Write Delimited Spreadsheet.vi"("file path (dialog if empty)"=w727, "2D data"=w728, "append to file? (new file:F)"=TRUE, "transpose? (no:F)"=TRUE) -> ("new file path (Not A Path if cancelled)"=w723:path)  [unwired: 10 in, 1 out]
        n191 = call-poly <vilib>:"Write Delimited Spreadsheet.vi"("file path (dialog if empty)"=w723, "1D data"=string[] ["Mean", "Std. Dev."], "append to file? (new file:F)"=TRUE, "transpose? (no:F)"=FALSE) -> ("new file path (Not A Path if cancelled)"=w719:path)  [unwired: 10 in, 1 out]
        n192 = call-poly <vilib>:"Write Delimited Spreadsheet.vi"("file path (dialog if empty)"=w719, "1D data"=w709, "append to file? (new file:F)"=TRUE, "transpose? (no:F)"=FALSE) -> ()  [unwired: 10 in, 2 out]
        n193 = local write "Export"(FALSE) -> ()
      }
      frame "AutoExportRun" {
        # "For Auto Export also add mean waveform"
        # "Get mean Data into 1D array Shift register for waveform"
        # "Gate Number is just number of count measurements"
        # "time...using array size"
        n194 = Array Size(array=w768) -> (size(s)=w770:i32)
        n195 = for {
          N: w770 -> [_]
          tunnel: [w812] -> w767 mode=indexing
          i -> [w814]
          n196 = local read "ITD"() -> (w816:i32)
          n197 = Add(x=1, y=w814) -> (x+y=w815:i32)
          n198 = Multiply(x=w816, y=w815) -> (x*y=w812:i32)
        }
        n199 = flat-sequence {
          tunnel: w759 -> [w811]
          tunnel: [w807] -> w758
          frame #0 {
            n200 = local read "SS"() -> (w810:i32)
            n201 = Multiply(x=w811, y=w810) -> (x*y=w808:i32)
            n202 = local read "SP"() -> (w809:i32)
            n203 = Add(x=w809, y=w808) -> (x+y=w807:i32)
          }
        }
        n204 = call <vilib>:"Std Deviation and Variance.vi"("X"=w768) -> ("mean"=w762:dbl, "standard deviation"=w752:dbl)  [unwired: 1 in, 1 out]
        n205 = Build Array(w762, w752) -> (w765:dbl[])
        n206 = Number To Decimal String(number=w758) -> (decimal integer string=w757:string)  [unwired: 1 in]
        n207 = Build Array(w754, w767, w768) -> (w769:u32[][])
        n208 = Build Array (concatenate)(string[] ["Angle (deg)"], w757) -> (w755:string[])
        n209 = case shown="True" "Save All Gate Data" {
          tunnel: w769 -> [_ w805]
          tunnel: w765 -> [_ w792]
          tunnel: [w785 w791] -> w764
          tunnel: w760 -> [w785 w790]
          tunnel: w755 -> [_ w786]
          frame False {
          }
          frame True {
            # "time...using array size"
            n210 = call-poly <vilib>:"Write Delimited Spreadsheet.vi"("file path (dialog if empty)"=w790, "1D data"=w786, "append to file? (new file:F)"=TRUE, "transpose? (no:F)"=FALSE) -> ("new file path (Not A Path if cancelled)"=w789:path)  [unwired: 10 in, 1 out]
            n211 = call-poly <vilib>:"Write Delimited Spreadsheet.vi"("file path (dialog if empty)"=w789, "1D data"=string[] ["Gate  No.", "Time [ms]", "Counts"], "append to file? (new file:F)"=TRUE, "transpose? (no:F)"=FALSE) -> ("new file path (Not A Path if cancelled)"=w804:path)  [unwired: 10 in, 1 out]
            n212 = call-poly <vilib>:"Write Delimited Spreadsheet.vi"("file path (dialog if empty)"=w804, "2D data"=w805, "append to file? (new file:F)"=TRUE, "transpose? (no:F)"=TRUE) -> ("new file path (Not A Path if cancelled)"=w800:path)  [unwired: 10 in, 1 out]
            n213 = call-poly <vilib>:"Write Delimited Spreadsheet.vi"("file path (dialog if empty)"=w800, "1D data"=string[] ["Mean", "Std. Dev."], "append to file? (new file:F)"=TRUE, "transpose? (no:F)"=FALSE) -> ("new file path (Not A Path if cancelled)"=w796:path)  [unwired: 10 in, 1 out]
            n214 = call-poly <vilib>:"Write Delimited Spreadsheet.vi"("file path (dialog if empty)"=w796, "1D data"=w792, "append to file? (new file:F)"=TRUE, "transpose? (no:F)"=FALSE) -> ("new file path (Not A Path if cancelled)"=w791:path)  [unwired: 10 in, 1 out]
          }
        }
        n215 = local write "Export"(FALSE) -> ()
      }
      frame "AutoExportSweep" {
        w820 = 0
        w819 = 0.0
        # "Gate Number is just number \nof count measurements"
        # "For Auto Export also add mean waveform"
        # "Get mean Data into 1D array Shift register for waveform"
        # "time...using array size"
        # "time...using array size"
        n216 = Array Size(array=w842) -> (size(s)=w857:i32)
        n217 = for {
          N: w857 -> [_]
          tunnel: [w892] -> w849 mode=indexing
          i -> [w889]
          n218 = local read "SS"() -> (w893:i32)
          n219 = Multiply(x=w893, y=w889) -> (x*y=w890:i32)
          n220 = local read "SP"() -> (w891:i32)
          n221 = Add(x=w891, y=w890) -> (x+y=w892:i32)
        }
        n222 = call <vilib>:"Std Deviation and Variance.vi"("X"=w842) -> ("mean"=w843:dbl, "standard deviation"=w837:dbl)  [unwired: 1 in, 1 out]
        n223 = Initialize Array(w819, w820) -> (w840:dbl[])
        n224 = Initialize Array(w819, w820) -> (w839:dbl[])
        n225 = Build Array(w843, w837) -> (w833:dbl[])
        n226 = Initialize Array(cluster{i32, i32} {0, 0}, w820) -> (w818:cluster{i32, i32}[])
        n227 = Build Array(w849, w842, w838) -> (w855:dbl[][])
        n228 = local read "RN"() -> (w825:i32)
        n229 = Number To Decimal String(number=w825) -> (decimal integer string=w824:string)  [unwired: 1 in]
        n230 = local read "IT"() -> (w823:i32)
        n231 = Number To Decimal String(number=w823) -> (decimal integer string=w822:string)  [unwired: 1 in]
        n232 = Build Array("Sample Name", "Laser Power (mW)", w824, w822) -> (w821:string[])
        n233 = for {
          N: 4 -> [_]
          shift-right: [w877] -> w828
          shift-left: w831 -> [w878]
          tunnel: string[] ["#Sample", "#LaserPower (mW)", "#NumGates", "#GateTime (ms)"] -> [w873] mode=indexing
          tunnel: w821 -> [w872] mode=indexing
          n234 = Build Array(w873, w872) -> (w874:string[])
          n235 = call-poly <vilib>:"Write Delimited Spreadsheet.vi"("file path (dialog if empty)"=w878, "1D data"=w874, "append to file? (new file:F)"=TRUE, "transpose? (no:F)"=FALSE) -> ("new file path (Not A Path if cancelled)"=w877:path)  [unwired: 10 in, 1 out]
        }
        n236 = call-poly <vilib>:"Write Delimited Spreadsheet.vi"("file path (dialog if empty)"=w828, "1D data"=string[] ["Angle", "CountsMean", "CountsSTD"], "append to file? (new file:F)"=TRUE, "transpose? (no:F)"=FALSE) -> ("new file path (Not A Path if cancelled)"=w854:path)  [unwired: 10 in, 1 out]
        n237 = call-poly <vilib>:"Write Delimited Spreadsheet.vi"("file path (dialog if empty)"=w854, "2D data"=w855, "append to file? (new file:F)"=TRUE, "transpose? (no:F)"=TRUE) -> ("new file path (Not A Path if cancelled)"=w851:path)  [unwired: 10 in, 1 out]
        n238 = case shown="False" FALSE {
          tunnel: w851 -> [w879 w887]
          tunnel: w833 -> [_ w884]
          tunnel: [w879 w881] -> w832
          frame False {
          }
          frame True {
            n239 = call-poly <vilib>:"Write Delimited Spreadsheet.vi"("file path (dialog if empty)"=w887, "1D data"=string[] ["Mean", "Std. Dev."], "append to file? (new file:F)"=TRUE, "transpose? (no:F)"=FALSE) -> ("new file path (Not A Path if cancelled)"=w885:path)  [unwired: 10 in, 1 out]
            n240 = call-poly <vilib>:"Write Delimited Spreadsheet.vi"("file path (dialog if empty)"=w885, "1D data"=w884, "append to file? (new file:F)"=TRUE, "transpose? (no:F)"=FALSE) -> ("new file path (Not A Path if cancelled)"=w881:path)  [unwired: 10 in, 1 out]
          }
        }
        n241 = local write "Export"(FALSE) -> ()
      }
      frame "AutoSweep" {
        w900 = 0
        # "1. Create a file path (Send two strings, \"SetPosition\" and \"AutoCount|nit!\")\n2. Send to \"SetPosition\"\n2.1. Will create a Position Number Shift register\n2.2. Move stage to initial position, allow time to complete movement or add delay\n3. Send to \"AutoCount|nit!\"\n3.1. \"AutoCount|nit!\" is clone of \"Count|nit!\" but sends to \"AutoCheckNumber\", not \"CheckNumber\n3.1.1. \"AutoCheckNumber\" will check if end position, or run condition is met then send \"CountStop\" and \"ActiveSwitch\"\n3.1.2. \"AutoCheck Number\" will allow \"CountStop\" to be sent via Stop Boolean\n3.1.3. \"AutoCheckNumber\" will upon END of one run will run \"AutoExportRun\" to set file path\n3.1.3.1. \"AutoExportRun\" will add a data point to Mean Waveform after Count Stop\n3.1.4. \"AutoCheckNumber\" will upon END of sweep will run \"AutoExportSweep\" then issue \"ActiveSwitch\"\n3.1.4.1. \"AutoExportSweep\" will append final Mean Sweep waveform to file path before \"CountStop\";\"ActiveSwitch\"\n4. If End condition not met; \"MotorJog\"; \"AutoCount|nit!\"....repeats\n4.1. Will move to next position by set increment, with .net code, add delay to allow it to arrive at position"
        # "Create a File path here\nSend switch case string \"SetPosition\", which has a position number switch register"
        # "1.Position Set, create a file path\n2. Count|nit!---duplicate and create auto counter, add read sweep data for auto read\n2.0.1Checknumber end, change active switch to Auto export\n3. Auto Export ... need to make \n3.0.2Auto Export end, send to read sweep data (mean, stdev for per sweep)\n3.Export\n4.check end position, check end condition met\n5.met>end;not end >continue\n6. Jog motor\n7.repeat from 2."
        # "Create Motor Controls for setting Homing, Step size for angle, idle time(if required),"
        n242 = local write "SN"(w900) -> ()
        n243 = call-poly <vilib>:"Write Delimited Spreadsheet.vi"("append to file? (new file:F)"=FALSE) -> ("new file path (Not A Path if cancelled)"=w899:path)  [unwired: 13 in, 1 out]
        n244 = Build Array("SetPosition", "AutoCount|nit!") -> (w905:string[])
        n245 = Build Array (concatenate)(w903, w905) -> (w902:string[])
        n246 = Wait (ms)(milliseconds to wait="Wait to Start (ms)") -> ()  [unwired: 1 out]
      }
      frame "MotorJog" {
        # "Move position by set increment"
        # "Add a test Jog?"
        # "Put thor labs net code here"
        n247 = stacked-sequence {
          tunnel: w932 -> [w954 w959]
          frame #0 {
            n248 = local read "SSD"() -> (w953:i32)
            n249 = invoke class="KCubeDCServo" method="MoveRelative"(reference=w954, "direction"=1, "stepSize"=w953, "waitTimeout"=0) -> ()  [unwired: 2 in, 6 out]
            n250 = local read "WT"() -> (w951:i32)
            n251 = Wait (ms)(milliseconds to wait=w951) -> ()  [unwired: 1 out]
          }
          frame #1 {
            n252 = invoke class="KCubeDCServo" method="GetPositionCounter"(reference=w959) -> ("GetPositionCounter"=w957:i32)  [unwired: 2 in, 2 out]
            n253 = Divide(x=w957, y=1919.6418578623338) -> (x/y=w955:dbl)
            n254 = Wait (ms)(milliseconds to wait=50) -> ()  [unwired: 1 out]
            n255 = local write "PC"(w955) -> ()
          }
        }
        n256 = local write "P8"(FALSE) -> ()
      }
      frame "SetPosition" {
        n257 = stacked-sequence {
          tunnel: w967 -> [w986 w989 w994]
          frame #0 {
            n258 = local read "SPD"() -> (w985:i32)
            n259 = invoke class="KCubeDCServo" method="SetMoveAbsolutePosition"(reference=w986, "position"=w985) -> ()  [unwired: 2 in, 4 out]
          }
          frame #1 {
            n260 = invoke class="KCubeDCServo" method="MoveAbsolute"(reference=w989, "waitTimeout"=0) -> ()  [unwired: 2 in, 4 out]
            n261 = local read "WT"() -> (w988:i32)
            n262 = Wait (ms)(milliseconds to wait=w988) -> ()  [unwired: 1 out]
          }
          frame #2 {
            n263 = invoke class="KCubeDCServo" method="GetPositionCounter"(reference=w994) -> ("GetPositionCounter"=w991:i32)  [unwired: 2 in, 2 out]
            n264 = Divide(x=w991, y=1919.6418578623338) -> (x/y=w990:dbl)
            n265 = local write "PC"(w990) -> ()
            n266 = Wait (ms)(milliseconds to wait=50) -> ()  [unwired: 1 out]
          }
        }
      }
      frame "", "Idle" {
        n267 = event shown="[12] \"Auto-Sweep\": Value Change" {
          selector: _ -> [_ _ _ _ _ _ _ _ _ _ _ _ _]
          dyn-events: _ -> [_ _ _ _ _ _ _ _ _ _ _ _ _]
          timeout: _ -> [_ _ _ _ _ _ _ _ _ _ _ _ _]
          tunnel: w1009 -> [w1024 w1027 w1030 w1034 w1038 w1042 w1046 w1050 w1053 w1055 w1058 w1061 w1064]
          tunnel: [w1022 w1026 w1029 w1033 w1037 w1041 w1045 w1049 w1052 w1054 w1057 w1060 w1065] -> w1007
          event Menu Selection (User) {
            n268 = event-data() -> ("ItemTag"=w1023:string)  [unwired: 1 out]
            n269 = Build Array (concatenate)(w1024, w1023) -> (w1022:string[])
          }
          event "EXIT": Value Change {
            n270 = event-data() -> ()  [unwired: 7 out]
            n271 = Build Array (concatenate)(w1027, "Exit") -> (w1026:string[])
          }
          event "P1": Value Change {
            n272 = event-data() -> ()  [unwired: 7 out]
            n273 = Build Array (concatenate)(w1030, "SetPower") -> (w1029:string[])
          }
          event "P2": Value Change {
            n274 = event-data() -> ()  [unwired: 7 out]
            n275 = Build Array (concatenate)(w1034, "ReadPower") -> (w1033:string[])
            n276 = Wait (ms)(milliseconds to wait=u32 200 ("ミリ秒待機時間")) -> ()  [unwired: 1 out]
          }
          event "P3": Value Change {
            n277 = event-data() -> ()  [unwired: 7 out]
            n278 = Build Array (concatenate)(w1038, "SetIT") -> (w1037:string[])
            n279 = Wait (ms)(milliseconds to wait=u32 200 ("ミリ秒待機時間")) -> ()  [unwired: 1 out]
          }
          event "P4": Value Change {
            n280 = event-data() -> ()  [unwired: 7 out]
            n281 = Build Array (concatenate)(w1042, "ReadIT") -> (w1041:string[])
            n282 = Wait (ms)(milliseconds to wait=u32 200 ("ミリ秒待機時間")) -> ()  [unwired: 1 out]
          }
          event "P5": Value Change {
            n283 = event-data() -> ()  [unwired: 7 out]
            n284 = Build Array (concatenate)(w1046, "SetRN") -> (w1045:string[])
            n285 = Wait (ms)(milliseconds to wait=u32 200 ("ミリ秒待機時間")) -> ()  [unwired: 1 out]
          }
          event "P6": Value Change {
            n286 = event-data() -> ()  [unwired: 7 out]
            n287 = Build Array (concatenate)(w1050, "ReadRN") -> (w1049:string[])
            n288 = Wait (ms)(milliseconds to wait=u32 200 ("ミリ秒待機時間")) -> ()  [unwired: 1 out]
          }
          event "Start": Value Change {
            n289 = event-data() -> ()  [unwired: 7 out]
            n290 = Build Array (concatenate)(w1053, "CountInit") -> (w1052:string[])
          }
          event "Export": Value Change {
            n291 = event-data() -> ()  [unwired: 7 out]
            n292 = Build Array (concatenate)(w1055, "Export") -> (w1054:string[])
          }
          event "P7": Value Change {
            n293 = event-data() -> ()  [unwired: 7 out]
            n294 = Build Array (concatenate)(w1058, "SetStepProp") -> (w1057:string[])
          }
          event "P8": Value Change {
            n295 = event-data() -> ()  [unwired: 7 out]
            n296 = Build Array (concatenate)(w1061, "MotorJog") -> (w1060:string[])
          }
          event "Auto-Sweep": Value Change {
            n297 = event-data() -> ()  [unwired: 7 out]
            n298 = Build Array (concatenate)(w1064, "AutoSweep") -> (w1065:string[])
            n299 = Wait (ms)(milliseconds to wait=200) -> ()  [unwired: 1 out]
          }
        }
        n300 = Build Array (concatenate)("", w1007) -> (w1006:string[])
      }
      frame "Error", Default {
        n301 = Concatenate Strings("Error  Case Name .....", "\r\n", w1077) -> (w1079:string)
        n302 = One Button Dialog(message=w1079) -> (true=w1078:bool)  [unwired: 1 out]
        n303 = stacked-sequence {
          tunnel: w1078 -> [_]
          frame #0 {
            n304 = Stop() -> ()  [unwired: 1 out]
          }
        }
      }
      frame "Exit" {
        # "See you again ......"
        n305 = call "Close.vi"("Handle"=w1106) -> ()  [unwired: 9 in, 2 out]
      }
    }
    n306 = Divide(x=w20, y=1919.6418578623338) -> (x/y=w15:dbl)
    n307 = local write "PC"(w15) -> ()
    n308 = call "SM_CaseErase.vi"("Input"=w45) -> ("Output"=w44:string[])  [unwired: 10 out]
  }
  n309 = invoke class="KCubeDCServoControl" method="CloseDevice"(reference=w7) -> ()  [unwired: 2 in, 3 out]
